vi "运维调试_五参数.vi"(11 "编号":string) -> ()   [LabVIEW 2016, in "斯坦道多参数.lvlib"]
uses:
  <vilib>/Utility/miscctls.llb/LVPointTypeDef.ctl
  <vilib>/Plasmionique/MB Master/MB_Master/MB_Master.lvclass
  <vilib>/Utility/config.llb/NI_LVConfig.lvlib
panel:
  in  "水样保存组数":dbl caption="水样保存组数:"
  in  "打开modbus":bool
  in  "仪器参数":bool
  in  "参数设置选项卡":enum32{"选项卡 1", "选项卡 2"}(tab)
  in  "pH":bool
  in  "DO":bool
  in  "Turb":bool
  in  "Cond":bool
  in  "Temp":bool
  in  "叶绿素a启用":bool
  in  "藻密度":bool
  in  "pH探头选择":u16(ring) items=["YL型", "MQ型", "NAQ型"]
  in  "DO探头选择":u16(ring) items=["YL型", "MQ型", "NAQ型"]
  in  "电导率探头选择":u16(ring) items=["YL型", "MQ型", "NAQ型"]
  in  "浊度探头选择":u16(ring) items=["YL型", "MQ型", "NAQ型"]
  in  "叶绿素a探头选择":u16(ring) items=["YL型", "MQ型", "NAQ型"]
  in  "藻密度探头选择":u16(ring) items=["YL型", "MQ型", "NAQ型"]
  in  "ORP启用":bool
  in  "ORP探头选择":u16(ring) items=["YL型", "MQ型", "NAQ型"]
  in  "校准选择":T1
  out "模块版本号":string
  out "权限等级":string
  in  "水样稳定时间":dbl caption="水样稳定时间:"
  out "选项卡控件":enum32{"选项卡 1", "选项卡 2"}(tab)
  in  "VISA资源名称":refnum<visa-resource-name> caption="串口"
  in  "电导率串口":refnum<visa-resource-name>
  in  "IP":string="localhost" caption="IP:"
  in  "Port":u16=502 caption="Port:"
  in  "自动断线重连":bool=TRUE
  in  "连接方式":u16(ring) items=["Modbus RTU", "Modbus TCP"]
  in  "密码锁":bool
  in  "设置页返回":bool
  in  "周期设置":bool
  out "当前串口":string
  out "运行状态":enum16{"空闲", "水样测试", "标样核查"}(ring)
  in  "停止":bool
  in  "标样核查":bool
  in  "水样测试":bool
  in  "设置":bool
  in  "探头校正返回":bool
  in  "探头校正":bool
  out "检测值":T2
  # "请设置仪器连接方式"
  # "组"
  # "请选择要启用的参数"
  # "min"
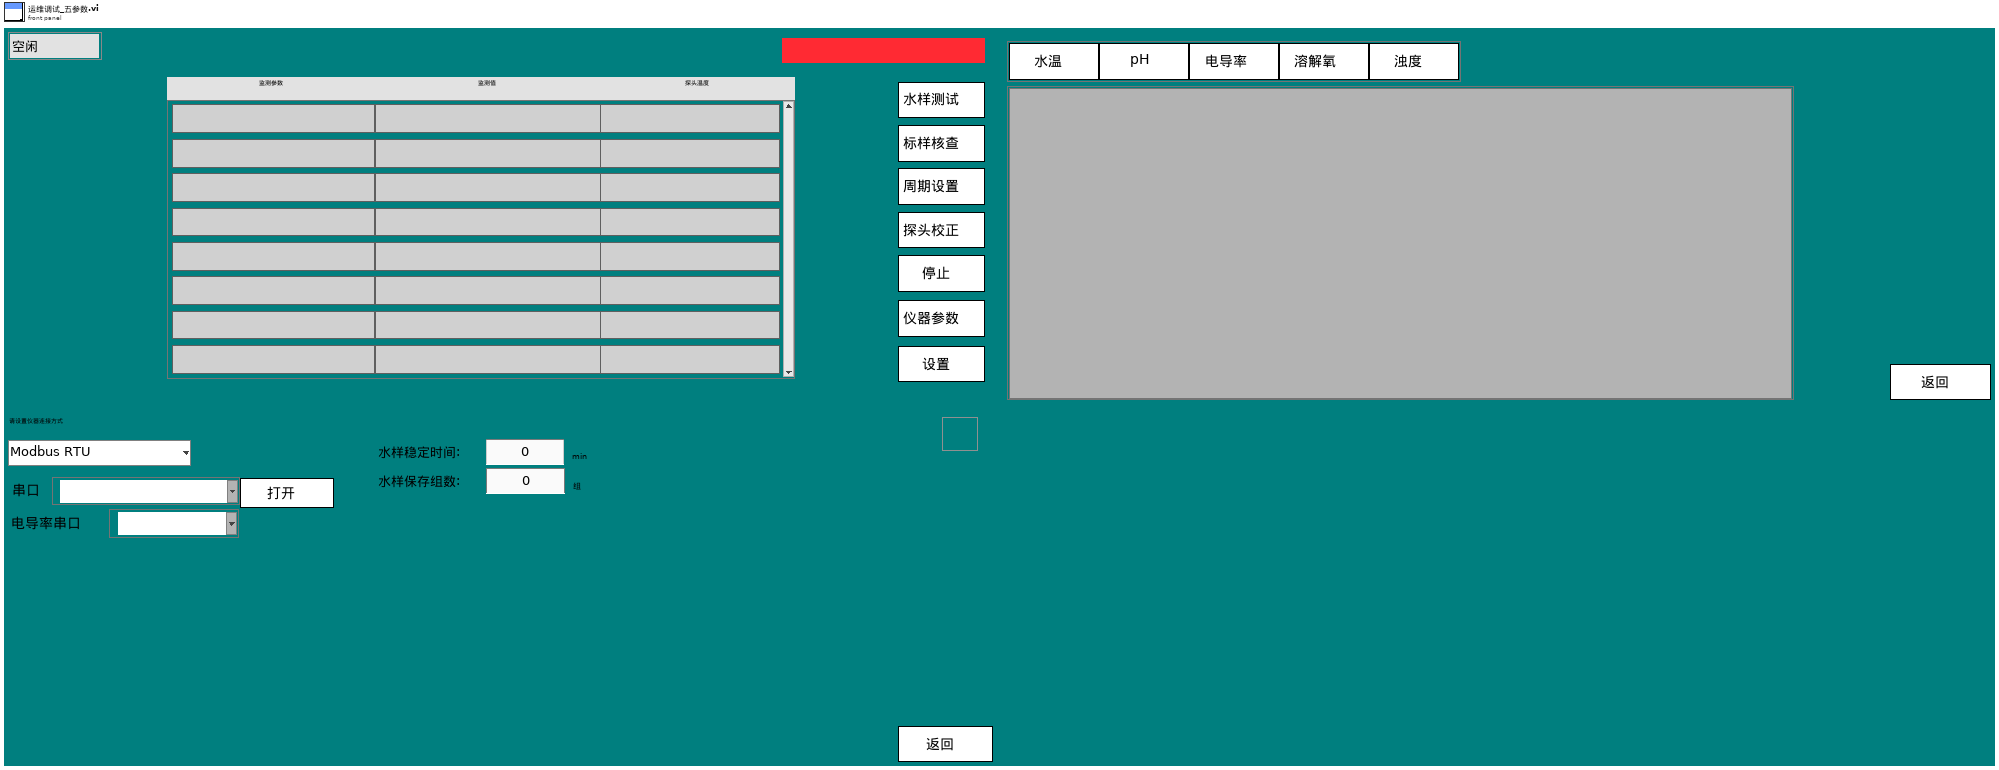
[diagram p1: front panel]
types:
  T1 = cluster{"水温校准":bool, "pH校准":bool, "电导率校准":bool, "溶解氧校准":bool, "浊度校准":bool, "叶绿素a校准":bool, "藻密度校准":bool, "ORP校准":bool}
  T2 = typedef "斯坦道多参数.lvlib/检测值.ctl" = cluster{"监测参数1":string, "浓度1":string, "探头温度1":string}[]
  T3 = typedef "LVPointTypeDef.ctl" = cluster{"Horizontal":i16, "Vertical":i16}
  T4 = cluster{"CH":u16, "监测值":dbl, "温度偏移修正值":sgl, "信号值":sgl}
  T5 = cluster{"温度测量值":sgl, "测量值":sgl, "温度偏移修正值":sgl, "信号值":sgl}
  T6 = cluster{"温度测量值":sgl, "DO%":sgl, "DOmg/L":sgl, "温度偏移修正值":sgl}
  T7 = cluster{"电极状态标志":u16, "电极型号标志":u16, "浊度测量值":sgl, "温度测量值":sgl, "浊度信号值":sgl, "浊度偏移修正值":sgl, "温度偏移修正值":sgl, "手动温度补偿值":sgl, "浊度电极零点":sgl, "浊度电极斜率":sgl, "第1点标准值记录":sgl, "第1点信号值记录":sgl, "第1点温度值记录":sgl, "第2点标准值记录":sgl, "第2点信号值记录":sgl, "第2点温度值记录":sgl, "命令滤波设定":u16, "温度模式":enum16{"ATC", "MTC"}, "生产批次":u16, "电极序号":u16, "串口地址":u16, "串口波特率":enum16{"9600", "19200", "115200"}, "串口校验位":enum16{"NONE", "ODD", "EVEN"}, "串口停止位":enum16{"1bit", "2bit"}, "第一点标准值":sgl, "第二点标准值":sgl, "第三点标准值":sgl}
  T8 = cluster{"电极状态标志":u16, "电极型号标志":u16, "溶解氧测量值":sgl, "温度测量值":sgl, "溶解氧饱和度值":sgl, "盐度补偿值":sgl, "大气压补偿值":sgl, "溶解氧偏移修正值":sgl, "温度偏移修正值":sgl, "手动温度补偿值":sgl, "溶解氧电极零点":sgl, "溶解氧电极斜率":sgl, "第1点标准值记录":sgl, "第1点信号值记录":sgl, "第1点温度值记录":sgl, "第2点标准值记录":sgl, "第2点信号值记录":sgl, "第2点温度值记录":sgl, "命令滤波设定":u16, "温度模式":enum16{"ATC", "MTC"}, "生产批次":u16, "电极序号":u16, "串口地址":u16, "串口波特率":enum16{"9600", "19200", "115200"}, "串口校验位":enum16{"NONE", "ODD", "EVEN"}, "串口停止位":enum16{"1bit", "2bit"}, "第一点标准值":sgl, "第二点标准值":sgl}
  T9 = cluster{"电极状态标志":u16, "电极型号标志":u16, "酸碱度测量值":sgl, "温度测量值":sgl, "酸碱度信号值":sgl, "温度信号值":sgl, "酸碱度偏移修正值":sgl, "温度偏移修正值":sgl, "手动温度补偿值":sgl, "酸碱度电极零点":sgl, "酸碱度电极斜率":sgl, "第1点标准值记录":sgl, "第1点信号值记录":sgl, "第1点温度值记录":sgl, "第2点标准值记录":sgl, "第2点信号值记录":sgl, "第2点温度值记录":sgl, "命令滤波设定":u16, "温度模式":enum16{"ATC", "MTC"}, "生产批次":u16, "电极序号":u16, "串口地址":u16, "串口波特率":enum16{"9600", "19200", "115200"}, "串口校验位":enum16{"NONE", "ODD", "EVEN"}, "串口停止位":enum16{"1bit", "2bit"}, "第一点标准值":sgl, "第二点标准值":sgl}
  T10 = cluster{"测量量程":dbl, "测量精度":dbl, "测量间隔":dbl, "消解温度":dbl, "消解时长":dbl, "空白校准时间":timestamp, "曲线截距":dbl, "曲线斜率":dbl, "测量检出限":dbl, "测量信号值":dbl, "线性相关系数":dbl, "二次多项式系数":dbl, "标样校准时间":timestamp, "稀释倍数":dbl, "三项式系数":dbl, "空白标定系数":dbl, "量程系数":dbl, "F0/ORPA":dbl, "F1/ORPB":dbl, "F2/ORPK":dbl, "F3":dbl, "F4":dbl, "F5":dbl, "F6":dbl, "F7":dbl, "X0/滴定数":dbl, "量程":dbl}
  T11 = cluster{"电极状态标志":u16, "电极型号标志":u16, "电导率测量值":sgl, "温度测量值":sgl, "电导率信号值":sgl, "温度信号值":sgl, "温度补偿系数":sgl, "电导率偏移修正值":sgl, "温度偏移修正值":sgl, "手动温度补偿值":sgl, "电导率电极零点":sgl, "电导率电极斜率":sgl, "命令滤波设定":u16, "温度模式":enum16{"ATC", "MTC"}, "生产批次":u16, "电极序号":u16, "串口地址":u16, "串口波特率":enum16{"9600", "19200", "115200"}, "串口校验位":enum16{"NONE", "ODD", "EVEN"}, "串口停止位":enum16{"1bit", "2bit"}, "第一点标准值":sgl, "第二点标准值":sgl}
  T12 = enum8{"Enabled", "Disabled", "Disabled and Grayed Out"}
  T13 = cluster{"pH探头选择":u16, "DO探头选择":u16, "电导率探头选择":u16, "浊度探头选择":u16, "叶绿素a探头选择":u16, "蓝绿藻探头选择":u16, "orp探头选择":u16}
  T14 = cluster{"监测参数1":string, "浓度1":string, "探头温度1":string}[]
  T15 = cluster{"周期设置类型":enum16{"定点启动", "间隔启动"}, "定时功能启用":bool, "定时间隔":u32, "24H周期设置":bool[]}
  T16 = enum32{"Bad", "Idle", "Run top level", "Running"}
  T17 = typedef "LVDateTimeRec.ctl" = cluster{"秒数的小数部分":dbl, "秒":i32, "分":i32, "时":i32, "日":i32, "月":i32, "年":i32, "天数（周）":i32, "天数（年）":i32, "DST":i32}
  T18 = cluster{"Major":u16, "Minor":u16, "Fix":u16, "Build":u16}
  T19 = typedef "NI_LVConfig.lvlib/Config Data RefNum.ctl" = refnum<k1>
  T20 = cluster{"baud rate (bps)":u32, "stop bits":u16, "parity":u16, "flow control":u16, "timeout":u32, "retries":i32}
  T21 = cluster{"pH校准VI引用句柄":refnum<vi>, "DO校准VI引用句柄":refnum<vi>, "COND校准VI引用句柄":refnum<vi>, "TURB校准VI引用句柄":refnum<vi>, "CHLA校准VI引用句柄":refnum<vi>, "BGA校准VI引用句柄":refnum<vi>, "ORP校准VI引用句柄":refnum<vi>}
  T22 = cluster{"测量量程":dbl, "测量精度":dbl, "测量间隔":dbl, "消解温度":dbl, "消解时长":dbl, "空白校准时间":timestamp, "曲线截距":dbl, "曲线斜率":dbl, "测量检出限":dbl, "测量信号值":dbl, "线性相关系数":dbl, "二次多项式系数":dbl, "标样校准时间":timestamp, "稀释倍数":dbl, "三项式系数":dbl, "空白标定系数":dbl, "量程系数":dbl, "F0/ORPA":dbl, "F1/ORPB":dbl, "F2/ORPK":dbl, "F3":dbl, "F4":dbl, "F5":dbl, "F6":dbl, "F7":dbl, "X0/滴定数":dbl, "量程":dbl}[]
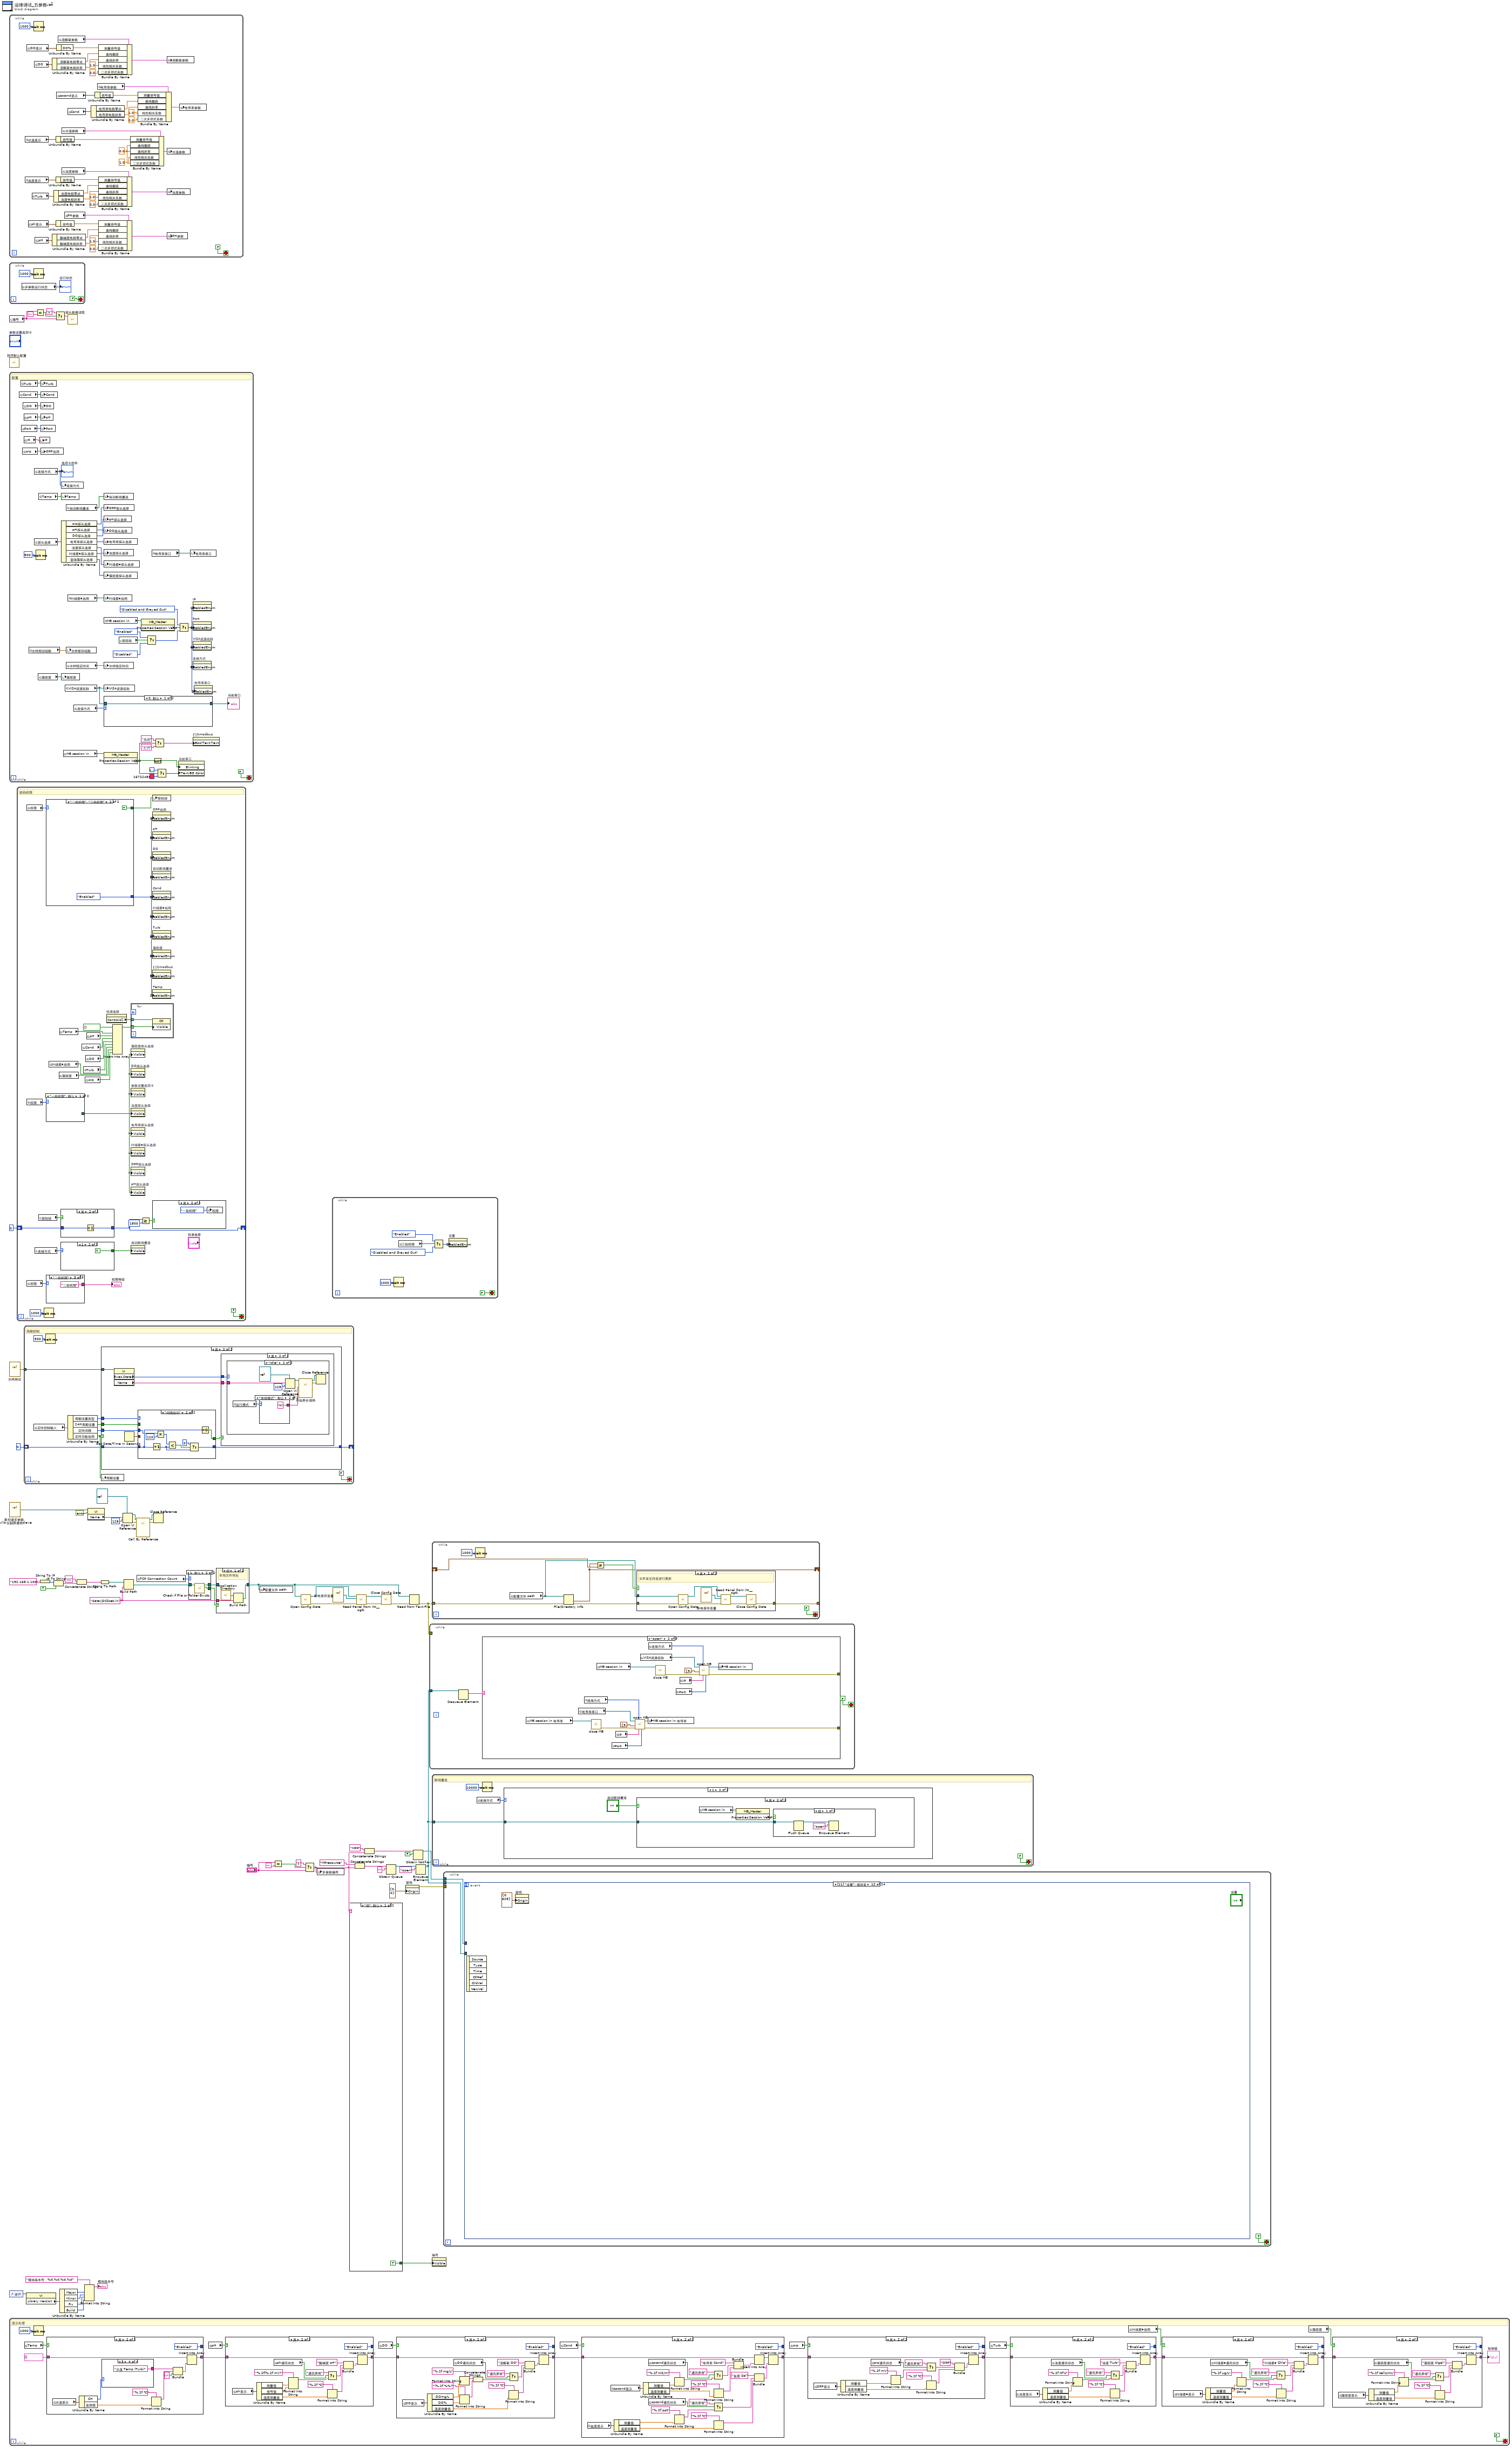
[diagram p0: block diagram]
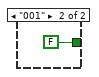
[diagram p3: hidden frame]
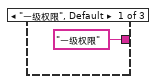
[diagram p12: hidden frame]
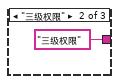
[diagram p13: hidden frame]
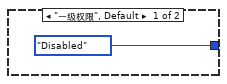
[diagram p14: hidden frame]
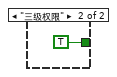
[diagram p15: hidden frame]
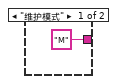
[diagram p19: hidden frame]
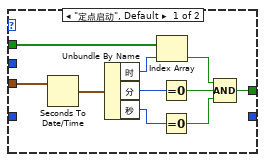
[diagram p20: hidden frame]
diagram:
  w34 = "data\\DCSset.ini" ("名称或相对路径")
  n1 = while {
    stop <- FALSE stop-if-true
    w64 = 0.0 ("二次多项式系数")
    n2 = global read "多参数全局变量.vi" "水温显示"() -> (w85:T4)
    n3 = global read "多参数全局变量.vi" "浊度显示"() -> (w67:T5)
    n4 = global read "多参数全局变量.vi" "DO显示"() -> (w99:T6)
    n5 = global read "多参数全局变量.vi" "ph显示"() -> (w94:T5)
    n6 = global read "国弘过程全局变量.vi" "Turb"() -> (w69:T7)
    n7 = Wait (ms)(milliseconds to wait=u32 1000 ("等待时间（毫秒）")) -> ()  [unwired: 1 out]
    n8 = global read "国弘过程全局变量.vi" "DO"() -> (w101:T8)
    n9 = global read "国弘过程全局变量.vi" "pH"() -> (w92:T9)
    n10 = Unbundle By Name(w101) -> ("溶解氧电极零点"=w102:sgl, "溶解氧电极斜率"=w103:sgl)
    n11 = Unbundle By Name(w92) -> ("酸碱度电极零点"=w91:sgl, "酸碱度电极斜率"=w90:sgl)
    n12 = Unbundle By Name(w69) -> ("浊度电极零点"=w70:sgl, "浊度电极斜率"=w71:sgl)
    n13 = Unbundle By Name(w85) -> ("信号值"=w86:sgl)
    n14 = Unbundle By Name(w67) -> ("信号值"=w68:sgl)
    n15 = Unbundle By Name(w94) -> ("信号值"=w93:sgl)
    n16 = Unbundle By Name(w99) -> ("DO%"=w100:sgl)
    n17 = global read "多参数全局变量.vi" "spcond显示"() -> (w80:T5)
    n18 = global read "断电保存变量.vi" "溶解氧参数"() -> (w97:T10)
    n19 = global read "断电保存变量.vi" "水温参数"() -> (w83:T10)
    n20 = global read "断电保存变量.vi" "浊度参数"() -> (w65:T10)
    n21 = global read "断电保存变量.vi" "PH参数"() -> (w96:T10)
    n22 = global read "国弘过程全局变量.vi" "Cond"() -> (w78:T11)
    n23 = Unbundle By Name(w78) -> ("电导率电极零点"=w77:sgl, "电导率电极斜率"=w76:sgl)
    n24 = Unbundle By Name(w80) -> ("信号值"=w79:sgl)
    n25 = global read "断电保存变量.vi" "电导率参数"() -> (w82:T10)
    n26 = Bundle By Name(cluster=w97, "测量信号值"=w100, "曲线截距"=w102, "曲线斜率"=w103, "线性相关系数"=1.0, "二次多项式系数"=0.0) -> (w98:T10)
    n27 = Bundle By Name(cluster=w65, "测量信号值"=w68, "曲线截距"=w70, "曲线斜率"=w71, "线性相关系数"=1.0, "二次多项式系数"=0.0) -> (w66:T10)
    n28 = Bundle By Name(cluster=w96, "测量信号值"=w93, "曲线截距"=w91, "曲线斜率"=w90, "线性相关系数"=1.0, "二次多项式系数"=0.0) -> (w95:T10)
    n29 = Bundle By Name(cluster=w83, "测量信号值"=w86, "曲线截距"=w64, "曲线斜率"=w64, "线性相关系数"=1.0, "二次多项式系数"=w64) -> (w84:T10)
    n30 = Bundle By Name(cluster=w82, "测量信号值"=w79, "曲线截距"=w77, "曲线斜率"=w76, "线性相关系数"=1.0, "二次多项式系数"=0.0) -> (w81:T10)
    n31 = global write "断电保存变量.vi" "溶解氧参数"(w98) -> ()
    n32 = global write "断电保存变量.vi" "水温参数"(w84) -> ()
    n33 = global write "断电保存变量.vi" "浊度参数"(w66) -> ()
    n34 = global write "断电保存变量.vi" "PH参数"(w95) -> ()
    n35 = global write "断电保存变量.vi" "电导率参数"(w81) -> ()
  }
  n36 = while {
    stop <- FALSE stop-if-true
    n37 = global read "多参数全局变量.vi" "多参数运行状态"() -> (→"运行状态":u16)
    n38 = Wait (ms)(milliseconds to wait=u32 1000 ("等待时间（毫秒）")) -> ()  [unwired: 1 out]
  }
  n39 = local read "编号"() -> (w10:string)
  n40 = call "程序默认配置.vi"() -> ()  [unwired: 11 in, 1 out]
  n41 = while {
    stop <- FALSE stop-if-true
    # "配置"
    n42 = global read "断电保存变量.vi" "Cond"() -> (w151:bool)
    n43 = global read "断电保存变量.vi" "Turb"() -> (w150:bool)
    n44 = global read "断电保存变量.vi" "Port"() -> (w129:u16)
    n45 = global read "断电保存变量.vi" "orp"() -> (w115:bool)
    n46 = global read "断电保存变量.vi" "DO"() -> (w152:bool)
    n47 = global read "断电保存变量.vi" "pH"() -> (w153:bool)
    n48 = global read "断电保存变量.vi" "IP"() -> (w130:string)
    n49 = global read "断电保存变量.vi" "水样测试组数"() -> (w111:dbl)
    n50 = global read "断电保存变量.vi" "连接方式"() -> (w123:u16)
    "选项卡控件" <- w123
    n51 = global read "断电保存变量.vi" "探头选择"() -> (w140:T13)
    n52 = Wait (ms)(milliseconds to wait=u32 500 ("等待时间（毫秒）")) -> ()  [unwired: 1 out]
    n53 = global read "断电保存变量.vi" "藻密度"() -> (w148:bool)
    n54 = global read "断电保存变量.vi" "Temp"() -> (w154:bool)
    n55 = local write "IP"(w130) -> ()
    n56 = local write "Turb"(w150) -> ()
    n57 = local write "Cond"(w151) -> ()
    n58 = local write "DO"(w152) -> ()
    n59 = local write "pH"(w153) -> ()
    n60 = local write "Port"(w129) -> ()
    n61 = local write "ORP启用"(w115) -> ()
    n62 = local write "连接方式"(w123) -> ()
    n63 = local write "Temp"(w154) -> ()
    n64 = Unbundle By Name(w140) -> ("orp探头选择"=w114:u16, "pH探头选择"=w124:u16, "DO探头选择"=w139:u16, "电导率探头选择"=w138:u16, "浊度探头选择"=w137:u16, "叶绿素a探头选择"=w136:u16, "蓝绿藻探头选择"=w135:u16)
    n65 = local write "藻密度"(w148) -> ()
    n66 = global read "多参数全局变量.vi" "MB session in"() -> (w144:refnum<class "MB_Master.lvclass">)
    n67 = global read "断电保存变量.vi" "VISA资源名称"() -> (w127:refnum<visa-resource-name>)
    n68 = global read "断电保存变量.vi" "自动断线重连"() -> (w118:bool)
    n69 = local write "水样保存组数"(w111) -> ()
    n70 = global read "断电保存变量.vi" "水样稳定时间"() -> (w117:dbl)
    n71 = global read "断电保存变量.vi" "叶绿素a启用"() -> (w149:bool)
    n72 = global read "断电保存变量.vi" "连接方式"() -> (w128:u16)
    n73 = local write "自动断线重连"(w118) -> ()
    n74 = local write "ORP探头选择"(w114) -> ()
    n75 = local write "pH探头选择"(w124) -> ()
    n76 = local write "DO探头选择"(w139) -> ()
    n77 = local write "电导率探头选择"(w138) -> ()
    n78 = local write "浊度探头选择"(w137) -> ()
    n79 = local write "叶绿素a探头选择"(w136) -> ()
    n80 = local write "藻密度探头选择"(w135) -> ()
    n81 = local write "叶绿素a启用"(w149) -> ()
    n82 = global read "多参数全局变量.vi" "MB session in"() -> (w147:refnum<class "MB_Master.lvclass">)
    n83 = local write "水样稳定时间"(w117) -> ()
    n84 = local write "VISA资源名称"(w127) -> ()
    n85 = case shown="0, 默认" w128 {
      tunnel: w127 -> [w156 _]
      tunnel: [w156 w157] -> w126
      frame 0, Default {
      }
      frame 1 {
        n86 = global read "断电保存变量.vi" "Port"() -> (w158:u16)
        n87 = global read "断电保存变量.vi" "IP"() -> (w160:string)
        n88 = Format Into String(format string=":%d" ("格式字符串"), initial string=w160, w158) -> (resulting string=w157:string)  [unwired: 1 in, 1 out]
      }
    }
    "当前串口" <- w126
    n89 = property class="MB_Master"(reference=w144) -> ("Properties:Session Valid"=w122:bool)  [unwired: 1 in, 2 out]
    n90 = local read "密码锁"() -> (w134:bool)
    n91 = property class="MB_Master"(reference=w147) -> ("Properties:Session Valid"=w146:bool)  [unwired: 1 in, 2 out]
    n92 = Select(t=T12."Enabled" ("f"), s=w134, f=T12."Disabled") -> (s? t:f=w132:T12)
    n93 = global read "断电保存变量.vi" "电导率串口"() -> (w112:refnum<visa-resource-name>)
    n94 = Not(x=w122) -> (.not. x?=w125:bool)
    n95 = Select(t="关闭" ("布尔文本.文本"), s=w122, f="打开" ("布尔文本.文本")) -> (s? t:f=w141:string)
    n96 = Select(t=u32 16777216, s=w122, f=u32 16722483) -> (s? t:f=w119:u32)
    n97 = property on="当前串口" class="Str"("Blinking"=w125, "Text.BG Color"=w119) -> ()  [unwired: 2 in, 2 out]
    n98 = Select(t=T12."Disabled and Grayed Out" ("禁用"), s=w146, f=w132) -> (s? t:f=w113:T12)
    n99 = local write "电导率串口"(w112) -> ()
    n100 = property on="IP" class="Str"("DisabledEnum"=w113) -> ()  [unwired: 2 in, 2 out]
    n101 = property on="Port" class="DigNum (严格)"("DisabledEnum"=w113) -> ()  [unwired: 2 in, 2 out]
    n102 = property on="VISA资源名称" class="VISAName"("DisabledEnum"=w113) -> ()  [unwired: 2 in, 2 out]
    n103 = property on="连接方式" class="Ring (严格)"("DisabledEnum"=w113) -> ()  [unwired: 2 in, 2 out]
    n104 = property on="打开modbus" class="Bool"("BoolText.Text"=w141) -> ()  [unwired: 2 in, 2 out]
    n105 = property on="电导率串口" class="VISAName"("DisabledEnum"=w113) -> ()  [unwired: 2 in, 2 out]
  }
  n106 = vi-ref "水样测试.vi"() -> (w53:refnum<vi>)
  n107 = vi-ref "斯坦道多参数.lvlib:主副屏通信slave.vi"() -> (w35:refnum<vi>)
  n108 = control-ref of="本VI"() -> (w26:refnum<vi>)
  n109 = while {
    stop <- FALSE stop-if-true
    # "显示处理"
    n110 = global read "断电保存变量.vi" "Temp"() -> (w177:bool)
    n111 = Wait (ms)(milliseconds to wait=u32 1000 ("等待时间（毫秒）")) -> ()  [unwired: 1 out]
    n112 = case shown="真" w177 {
      tunnel: [w318 w323] -> w174
      tunnel: T14 [] ("数组") -> [w318 w324]
      tunnel: [T12."Disabled and Grayed Out" ("禁用") T12."Enabled" ("禁用")] -> _
      frame False {
      }
      frame True {
        n113 = global read "多参数全局变量.vi" "水温显示"() -> (w321:T4)
        n114 = Unbundle By Name(w321) -> ("CH"=w320:u16, "监测值"=w319:dbl)
        n115 = case shown="3" w320 {
          tunnel: ["水温 Temp (pH)" ("监测参数1") "水温 Temp (Cond)" ("监测参数1") "水温 Temp (DO)" ("监测参数1") "水温 Temp (Turb)" ("监测参数1")] -> w328
          frame 0, Default {
          }
          frame 1 {
          }
          frame 2 {
          }
          frame 3 {
          }
        }
        n116 = Format Into String(format string="%.2f ℃" ("格式字符串"), w319) -> (resulting string=w327:string)  [unwired: 2 in, 1 out]
        n117 = Bundle("监测参数1"=w328, w327, "探头温度1"="-") -> (w325:cluster{"监测参数1":string, string, "探头温度1":string})  [unwired: 1 in]
        n118 = Insert Into Array(array=w324, new element=w325) -> (w323:T14)  [unwired: 1 in]
      }
    }
    n119 = global read "断电保存变量.vi" "pH"() -> (w175:bool)
    n120 = case shown="真" w175 {
      tunnel: [w300 w308] -> w172
      tunnel: w174 -> [w300 w310]
      tunnel: [T12."Disabled and Grayed Out" ("禁用") T12."Enabled" ("禁用")] -> _
      frame False {
      }
      frame True {
        n121 = global read "多参数全局变量.vi" "ph显示"() -> (w306:T5)
        n122 = Unbundle By Name(w306) -> ("测量值"=w316:sgl, "信号值"=w301:sgl, "温度测量值"=w314:sgl)
        n123 = global read "多参数全局变量.vi" "ph通讯状态"() -> (w304:bool)
        n124 = Format Into String(format string="%.2f(%.2f mV)" ("格式字符串"), w316, w301) -> (resulting string=w303:string)  [unwired: 2 in, 1 out]
        n125 = Select(t="通讯异常" ("格式字符串"), s=w304, f=w303) -> (s? t:f=w302:string)
        n126 = Format Into String(format string="%.2f ℃" ("格式字符串"), w314) -> (resulting string=w312:string)  [unwired: 2 in, 1 out]
        n127 = Bundle("监测参数2"="酸碱度 pH", "格式字符串"=w302, w312) -> (w309:cluster{"监测参数2":string, "格式字符串":string, string})  [unwired: 1 in]
        n128 = Insert Into Array(array=w310, new element=w309) -> (w308:T14)  [unwired: 1 in]
      }
    }
    n129 = global read "断电保存变量.vi" "DO"() -> (w173:bool)
    n130 = case shown="真" w173 {
      tunnel: [w279 w286] -> w169
      tunnel: w172 -> [w279 w287]
      tunnel: [T12."Disabled and Grayed Out" ("禁用") T12."Enabled" ("禁用")] -> _
      frame False {
      }
      frame True {
        n131 = global read "多参数全局变量.vi" "DO显示"() -> (w284:T6)
        n132 = Unbundle By Name(w284) -> ("DOmg/L"=w295:sgl, "DO%"=w293:sgl, "温度测量值"=w297:sgl)
        n133 = global read "多参数全局变量.vi" "DO通讯状态"() -> (w282:bool)
        n134 = Format Into String(format string="%.2f mg/L" ("格式字符串"), w295) -> (resulting string=w292:string)  [unwired: 2 in, 1 out]
        n135 = Format Into String(format string="(%.2f %%)" ("格式字符串"), w293) -> (resulting string=w291:string)  [unwired: 2 in, 1 out]
        n136 = Concatenate Strings(w292, w291) -> (w281:string)
        n137 = Select(t="通讯异常" ("格式字符串"), s=w282, f=w281) -> (s? t:f=w280:string)
        n138 = Format Into String(format string="%.2f ℃" ("格式字符串"), w297) -> (resulting string=w289:string)  [unwired: 2 in, 1 out]
        n139 = Bundle("监测参数2"="溶解氧 DO", "格式字符串"=w280, w289) -> (w288:cluster{"监测参数2":string, "格式字符串":string, string})  [unwired: 1 in]
        n140 = Insert Into Array(array=w287, new element=w288) -> (w286:T14)  [unwired: 1 in]
      }
    }
    n141 = global read "断电保存变量.vi" "Cond"() -> (w171:bool)
    n142 = case shown="真" w171 {
      tunnel: w169 -> [w249 w273]
      tunnel: [w249 w262] -> w161
      tunnel: [T12."Disabled and Grayed Out" ("禁用") T12."Enabled" ("禁用")] -> _
      frame False {
      }
      frame True {
        n143 = global read "多参数全局变量.vi" "盐度显示"() -> (w255:T5)
        n144 = global read "多参数全局变量.vi" "spcond显示"() -> (w270:T5)
        n145 = Unbundle By Name(w255) -> ("测量值"=w256:sgl, "温度测量值"=w257:sgl)
        n146 = Unbundle By Name(w270) -> ("测量值"=w269:sgl, "温度测量值"=w268:sgl)
        n147 = global read "多参数全局变量.vi" "spcond通讯状态"() -> (w266:bool)
        n148 = global read "多参数全局变量.vi" "spcond通讯状态"() -> (w259:bool)
        n149 = Format Into String(format string="%.2f mS/m" ("格式字符串"), w269) -> (resulting string=w265:string)  [unwired: 2 in, 1 out]
        n150 = Format Into String(format string="%.2f ppt" ("格式字符串"), w256) -> (resulting string=w260:string)  [unwired: 2 in, 1 out]
        n151 = Select(t="通讯异常" ("格式字符串"), s=w266, f=w265) -> (s? t:f=w264:string)
        n152 = Select(t="通讯异常" ("格式字符串"), s=w259, f=w260) -> (s? t:f=w261:string)
        n153 = Format Into String(format string="%.2f ℃" ("格式字符串"), w268) -> (resulting string=w274:string)  [unwired: 2 in, 1 out]
        n154 = Format Into String(format string="%.2f ℃" ("格式字符串"), w257) -> (resulting string=w254:string)  [unwired: 2 in, 1 out]
        n155 = Bundle("监测参数2"="电导率 Cond", "格式字符串"=w264, w274) -> (w272:cluster{"监测参数2":string, "格式字符串":string, string})  [unwired: 1 in]
        n156 = Insert Into Array(array=w273, new element=w272) -> (w263:T14)  [unwired: 1 in]
        n157 = Bundle("监测参数2"="盐度 Sal", "格式字符串"=w261, w254) -> (w250:cluster{"监测参数2":string, "格式字符串":string, string})  [unwired: 1 in]
        n158 = Insert Into Array(array=w263, new element=w250) -> (w262:T14)  [unwired: 1 in]
      }
    }
    n159 = global read "断电保存变量.vi" "orp"() -> (w163:bool)
    n160 = case shown="真" w163 {
      tunnel: w161 -> [w181 w192]
      tunnel: [w181 w190] -> w162
      tunnel: [T12."Disabled and Grayed Out" ("禁用") T12."Enabled" ("禁用")] -> _
      frame False {
      }
      frame True {
        n161 = global read "多参数全局变量.vi" "ORP显示"() -> (w188:T5)
        n162 = Unbundle By Name(w188) -> ("测量值"=w187:sgl, "温度测量值"=w186:sgl)
        n163 = global read "多参数全局变量.vi" "orp通讯状态"() -> (w184:bool)
        n164 = Format Into String(format string="%.2f mV" ("格式字符串"), w187) -> (resulting string=w183:string)  [unwired: 2 in, 1 out]
        n165 = Select(t="通讯异常" ("格式字符串"), s=w184, f=w183) -> (s? t:f=w182:string)
        n166 = Format Into String(format string="%.2f ℃" ("格式字符串"), w186) -> (resulting string=w193:string)  [unwired: 2 in, 1 out]
        n167 = Bundle("监测参数2"="ORP", "格式字符串"=w182, w193) -> (w191:cluster{"监测参数2":string, "格式字符串":string, string})  [unwired: 1 in]
        n168 = Insert Into Array(array=w192, new element=w191) -> (w190:T14)  [unwired: 1 in]
      }
    }
    n169 = global read "断电保存变量.vi" "Turb"() -> (w170:bool)
    n170 = case shown="真" w170 {
      tunnel: w162 -> [w232 w243]
      tunnel: [w232 w241] -> w168
      tunnel: [T12."Disabled and Grayed Out" ("禁用") T12."Enabled" ("禁用")] -> _
      frame False {
      }
      frame True {
        n171 = global read "多参数全局变量.vi" "浊度显示"() -> (w239:T5)
        n172 = Unbundle By Name(w239) -> ("测量值"=w238:sgl, "温度测量值"=w237:sgl)
        n173 = global read "多参数全局变量.vi" "浊度通讯状态"() -> (w235:bool)
        n174 = Format Into String(format string="%.2f NTU" ("格式字符串"), w238) -> (resulting string=w234:string)  [unwired: 2 in, 1 out]
        n175 = Select(t="通讯异常" ("格式字符串"), s=w235, f=w234) -> (s? t:f=w233:string)
        n176 = Format Into String(format string="%.2f ℃" ("格式字符串"), w237) -> (resulting string=w245:string)  [unwired: 2 in, 1 out]
        n177 = Bundle("监测参数2"="浊度 Turb", "格式字符串"=w233, w245) -> (w242:cluster{"监测参数2":string, "格式字符串":string, string})  [unwired: 1 in]
        n178 = Insert Into Array(array=w243, new element=w242) -> (w241:T14)  [unwired: 1 in]
      }
    }
    n179 = global read "断电保存变量.vi" "叶绿素a启用"() -> (w167:bool)
    n180 = case shown="真" w167 {
      tunnel: w168 -> [w215 w226]
      tunnel: [w215 w224] -> w165
      tunnel: [T12."Disabled and Grayed Out" ("禁用") T12."Enabled" ("禁用")] -> _
      frame False {
      }
      frame True {
        n181 = global read "多参数全局变量.vi" "叶绿素a显示"() -> (w220:T5)
        n182 = Unbundle By Name(w220) -> ("测量值"=w223:sgl, "温度测量值"=w222:sgl)
        n183 = global read "多参数全局变量.vi" "叶绿素a通讯状态"() -> (w218:bool)
        n184 = Format Into String(format string="%.2f μg/L" ("格式字符串"), w223) -> (resulting string=w217:string)  [unwired: 2 in, 1 out]
        n185 = Select(t="通讯异常" ("格式字符串"), s=w218, f=w217) -> (s? t:f=w216:string)
        n186 = Format Into String(format string="%.2f ℃" ("格式字符串"), w222) -> (resulting string=w228:string)  [unwired: 2 in, 1 out]
        n187 = Bundle("监测参数2"="叶绿素a Chla", "格式字符串"=w216, w228) -> (w225:cluster{"监测参数2":string, "格式字符串":string, string})  [unwired: 1 in]
        n188 = Insert Into Array(array=w226, new element=w225) -> (w224:T14)  [unwired: 1 in]
      }
    }
    n189 = global read "断电保存变量.vi" "藻密度"() -> (w166:bool)
    n190 = case shown="真" w166 {
      tunnel: w165 -> [w198 w209]
      tunnel: [w198 w207] -> w164
      tunnel: [T12."Disabled and Grayed Out" ("禁用") T12."Enabled" ("禁用")] -> _
      frame False {
      }
      frame True {
        n191 = global read "多参数全局变量.vi" "藻密度显示"() -> (w203:T5)
        n192 = Unbundle By Name(w203) -> ("测量值"=w206:sgl, "温度测量值"=w205:sgl)
        n193 = global read "多参数全局变量.vi" "藻密度通讯状态"() -> (w201:bool)
        n194 = Format Into String(format string="%.2f cells/mL" ("格式字符串"), w206) -> (resulting string=w200:string)  [unwired: 2 in, 1 out]
        n195 = Select(t="通讯异常" ("格式字符串"), s=w201, f=w200) -> (s? t:f=w199:string)
        n196 = Format Into String(format string="%.2f ℃" ("格式字符串"), w205) -> (resulting string=w211:string)  [unwired: 2 in, 1 out]
        n197 = Bundle("监测参数2"="藻密度 Algal", "格式字符串"=w199, w211) -> (w208:cluster{"监测参数2":string, "格式字符串":string, string})  [unwired: 1 in]
        n198 = Insert Into Array(array=w209, new element=w208) -> (w207:T14)  [unwired: 1 in]
      }
    }
    "检测值" <- w164
  }
  n199 = while {
    shift-right: [w356] -> _
    shift-left: u32 0 ("等待时间（毫秒）") -> [w357]
    stop <- FALSE stop-if-true
    # "密码权限"
    n200 = global read "多参数全局变量.vi" "权限"() -> (w347:enum16{"一级权限", "二级权限", "三级权限"})
    n201 = global read "多参数全局变量.vi" "权限"() -> (w348:enum16{"一级权限", "二级权限", "三级权限"})
    n202 = global read "多参数全局变量.vi" "权限"() -> (w349:enum16{"一级权限", "二级权限", "三级权限"})
    n203 = local read "连接方式"() -> (w353:u16)
    n204 = local read "密码锁"() -> (w358:bool)
    n205 = Wait (ms)(milliseconds to wait=u32 1000 ("等待时间（毫秒）")) -> ()  [unwired: 1 out]
    n206 = case shown="\"二级权限\", \"三级权限\"" w347 {
      tunnel: [T12."Disabled" ("禁用") T12."Enabled" ("禁用")] -> w351
      tunnel: [_ TRUE ("可见")] -> w346
      frame "一级权限", Default {
      }
      frame "二级权限", "三级权限" {
      }
    }
    n207 = case shown="\"一级权限\", 默认" w348 {
      tunnel: [_ TRUE ("可见")] -> w334
      frame "一级权限", Default {
      }
      frame "三级权限" {
      }
    }
    n208 = case shown="\"二级权限\"" w349 {
      tunnel: ["一级权限" ("权限等级") "三级权限" ("权限等级") "二级权限" ("权限等级")] -> w350
      frame "一级权限", Default {
      }
      frame "三级权限" {
      }
      frame "二级权限" {
      }
    }
    "权限等级" <- w350
    n209 = global read "断电保存变量.vi" "叶绿素a启用"() -> (w338:bool)
    n210 = global read "断电保存变量.vi" "藻密度"() -> (w337:bool)
    n211 = global read "断电保存变量.vi" "Temp"() -> (w344:bool)
    n212 = case shown="真" w358 {
      tunnel: w357 -> [_ w366]
      tunnel: [_ w365] -> w356
      frame False {
      }
      frame True {
        n213 = Increment(x=w366) -> (x+1=w365:u32)
      }
    }
    n214 = case shown="1" w353 {
      tunnel: [_ TRUE ("可见")] -> w352
      frame 0, Default {
      }
      frame 1 {
      }
    }
    n215 = global read "断电保存变量.vi" "Cond"() -> (w341:bool)
    n216 = global read "断电保存变量.vi" "Turb"() -> (w339:bool)
    n217 = global read "断电保存变量.vi" "orp"() -> (w336:bool)
    n218 = global read "断电保存变量.vi" "DO"() -> (w340:bool)
    n219 = global read "断电保存变量.vi" "pH"() -> (w342:bool)
    n220 = property on="校准选择" class="Clust"() -> ("Controls[]"=w345:refnum<vi>[])  [unwired: 2 in, 2 out]
    n221 = Insert Into Array(array=bool[] [] ("数组"), new element #1=w344, new element #2=w342, new element #3=w341, new element #4=w340, new element #5=w339, new element #6=w338, new element #7=w337, new element #8=w336) -> (w335:bool[])  [unwired: 1 in]
    n222 = for {
      tunnel: w345 -> [w362] mode=indexing
      tunnel: w335 -> [w361] mode=indexing
      n223 = property class="Ctl"(reference=w362, "Visible"=w361) -> ()  [unwired: 1 in, 2 out]
    }
    n224 = property on="藻密度探头选择" class="Ring (严格)"("Visible"=w334) -> ()  [unwired: 2 in, 2 out]
    n225 = property on="DO探头选择" class="Ring (严格)"("Visible"=w334) -> ()  [unwired: 2 in, 2 out]
    n226 = property on="参数设置选项卡" class="TabCtl (严格)"("Visible"=w334) -> ()  [unwired: 2 in, 2 out]
    n227 = property on="浊度探头选择" class="Ring (严格)"("Visible"=w334) -> ()  [unwired: 2 in, 2 out]
    n228 = property on="电导率探头选择" class="Ring (严格)"("Visible"=w334) -> ()  [unwired: 2 in, 2 out]
    n229 = property on="叶绿素a探头选择" class="Ring (严格)"("Visible"=w334) -> ()  [unwired: 2 in, 2 out]
    n230 = property on="ORP探头选择" class="Ring (严格)"("Visible"=w334) -> ()  [unwired: 2 in, 2 out]
    n231 = property on="pH探头选择" class="Ring (严格)"("Visible"=w334) -> ()  [unwired: 2 in, 2 out]
    n232 = property on="自动断线重连" class="Bool (严格)"("Visible"=w352) -> ()  [unwired: 2 in, 2 out]
    n233 = Greater Or Equal?(x=w356, y=u32 1800) -> (x >= y?=w354:bool)
    n234 = local write "密码锁"(w346) -> ()
    n235 = property on="ORP启用" class="Bool (严格)"("DisabledEnum"=w351) -> ()  [unwired: 2 in, 2 out]
    n236 = property on="pH" class="Bool (严格)"("DisabledEnum"=w351) -> ()  [unwired: 2 in, 2 out]
    n237 = property on="DO" class="Bool (严格)"("DisabledEnum"=w351) -> ()  [unwired: 2 in, 2 out]
    n238 = property on="自动断线重连" class="Bool (严格)"("DisabledEnum"=w351) -> ()  [unwired: 2 in, 2 out]
    n239 = property on="Cond" class="Bool (严格)"("DisabledEnum"=w351) -> ()  [unwired: 2 in, 2 out]
    n240 = property on="叶绿素a启用" class="Bool (严格)"("DisabledEnum"=w351) -> ()  [unwired: 2 in, 2 out]
    n241 = property on="Turb" class="Bool (严格)"("DisabledEnum"=w351) -> ()  [unwired: 2 in, 2 out]
    n242 = property on="藻密度" class="Bool (严格)"("DisabledEnum"=w351) -> ()  [unwired: 2 in, 2 out]
    n243 = property on="打开modbus" class="Bool"("DisabledEnum"=w351) -> ()  [unwired: 2 in, 2 out]
    n244 = property on="Temp" class="Bool (严格)"("DisabledEnum"=w351) -> ()  [unwired: 2 in, 2 out]
    n245 = case shown="真" w354 {
      frame False {
      }
      frame True {
        n246 = global write "多参数全局变量.vi" "权限"(enum16{"一级权限", "二级权限", "三级权限"}."一级权限" ("权限")) -> ()
      }
    }
  }
  n247 = while {
    tunnel: w53 -> [w376]
    shift-right: [w375] -> _
    shift-left: u32 0 ("等待时间（毫秒）") -> [w377]
    stop <- FALSE stop-if-true
    # "周期控制"
    n248 = global read "断电保存变量.vi" "定时控制输入"() -> (w379:T15)
    n249 = Wait (ms)(milliseconds to wait=u32 500 ("等待时间（毫秒）")) -> ()  [unwired: 1 out]
    n250 = Unbundle By Name(w379) -> ("周期设置类型"=w381:enum16{"定点启动", "间隔启动"}, "24H周期设置"=w380:bool[], "定时间隔"=w378:u32, "定时功能启用"=w374:bool)
    n251 = case shown="真" w374 {
      tunnel: w381 -> [_ w392]
      tunnel: w380 -> [_ w391]
      tunnel: w378 -> [_ w389]
      tunnel: w377 -> [_ w385]
      tunnel: w376 -> [_ w388]
      tunnel: [_ w384] -> w375
      frame False {
      }
      frame True {
        n252 = property class="VI"(reference=w388) -> ("Exec.State"=w386:T16, "Name"=w387:string)  [unwired: 1 in, 2 out]
        n253 = Get Date/Time In Seconds() -> (seconds since 1Jan1904=w393:timestamp)
        n254 = case shown="\"间隔启动\"" w392 {
          tunnel: w393 -> [w415 _]
          tunnel: w391 -> [w412 _]
          tunnel: [w406 w423] -> w390
          tunnel: w389 -> [_ w422]
          tunnel: w385 -> [_ w424]
          tunnel: [_ w418] -> w384
          frame "定点启动", Default {
            n255 = Seconds To Date/Time(time stamp (now)=w415) -> (date time rec=w414:T17)  [unwired: 1 in]
            n256 = Unbundle By Name(w414) -> ("时"=w413:i32, "分"=w411:i32, "秒"=w410:i32)
            n257 = Index Array(array=w412, index=w413) -> (element=w409:bool)
            n258 = Equal To 0?(x=w411) -> (x = 0?=w408:bool)
            n259 = Equal To 0?(x=w410) -> (x = 0?=w407:bool)
            n260 = Compound Arithmetic op=AND ("复合运算")(w409, w408, w407) -> (w406:bool)
          }
          frame "间隔启动" {
            n261 = Increment(x=w424) -> (x+1=w417:u32)
            n262 = Multiply(x=w422, y=u32 120) -> (x*y=w416:u32)
            n263 = Less?(x=w416, y=w417) -> (x < y?=w420:bool)
            n264 = Select(t=u32 0 ("y"), s=w420, f=w417) -> (s? t:f=w418:u32)
            n265 = Equal To 0?(x=w424) -> (x = 0?=w423:bool)
          }
        }
        n266 = case shown="真" w390 {
          tunnel: w386 -> [_ w395]
          tunnel: w387 -> [_ w394]
          frame False {
          }
          frame True {
            n267 = case shown="\"Idle\"" w395 {
              tunnel: w394 -> [_ w400]
              frame "Bad", Default {
              }
              frame "Idle" {
                n268 = global read "多参数全局变量.vi" "运行模式"() -> (w398:enum16{"维护模式", "常规模式", "应急模式", "质控模式"})
                n269 = case shown="\"常规模式\", 默认" w398 {
                  tunnel: ["M" ("数据标记表") "N" ("数据标记表")] -> w397
                  frame "维护模式" {
                  }
                  frame "常规模式", Default {
                  }
                }
                n270 = Open VI Reference(type specifier VI Refnum (for type only)=refnum<vi> refnum, vi path=w400, options=128 ("选项")) -> (vi reference=w401:refnum<vi>)  [unwired: 3 in, 1 out]
                n271 = call-by-ref "开始异步调用"(reference=w401, "数据标记表"=w397) -> (reference out=w402:refnum<vi>, error out=w403:errorcluster)  [unwired: 12 in]
                n272 = Close Reference(reference=w402, error in (no error)=w403) -> ()  [unwired: 1 out]
              }
            }
          }
        }
      }
    }
    n273 = local write "周期设置"(w374) -> ()
  }
  n274 = property class="VI"(reference=w26) -> ("Library.Version"=w25:T18)  [unwired: 1 in, 2 out]
  n275 = Equal?(x=w10, y="") -> (x = y?=w12:bool)
  n276 = String To IP(1:"192.168.1.100" ("名称")) -> (0:w33:u32)
  n277 = IP To String(1:TRUE ("句点符号？(F)"), 2:w33) -> (0:w30:string)
  n278 = Select(t="1", s=w12, f=w10) -> (s? t:f=w9:string)
  n279 = Unbundle By Name(w25) -> ("Major"=w23:u16, "Minor"=w22:u16, "Fix"=w21:u16, "Build"=w20:u16)
  n280 = call "探头数据读取.vi"("编号"=w9) -> ()  [unwired: 11 in]
  n281 = Concatenate Strings("\\\\" ("字符串"), w30) -> (w31:string)
  n282 = Format Into String(format string="模块版本号：%d.%d.%d.%d" ("格式字符串"), w23, w22, w21, w20) -> (resulting string=→"模块版本号":string)  [unwired: 2 in, 1 out]
  n283 = property class="VI"(reference=w35, error in=errorcluster {"status"=FALSE, "code"=0, "source"=""} ("错误输出")) -> ("Name"=w36:string)  [unwired: 2 out]
  n284 = String To Path(string=w31) -> (path=w28:path)
  n285 = Open VI Reference(type specifier VI Refnum (for type only)=refnum<vi> refnum, vi path=w36, options=128 ("选项")) -> (vi reference=w38:refnum<vi>, error out=w40:errorcluster)  [unwired: 3 in]
  n286 = Build Path(base path=w28, name or relative path=w34) -> (appended path=w4:path)
  n287 = call-by-ref "?"(reference=w38, error in=w40) -> (reference out=w42:refnum<vi>, error out=w41:errorcluster)  [unwired: 12 in]
  n288 = global read "多参数全局变量.vi" "TCP Connection Count"() -> (w5:u32)
  n289 = Close Reference(reference=w42, error in (no error)=w41) -> ()  [unwired: 1 out]
  n290 = case shown="1, 默认" w5 {
    tunnel: w4 -> [w425 w428]
    tunnel: [w425 w427] -> w2
    tunnel: [_ w426] -> w3
    frame 0 {
    }
    frame 1, Default {
      n291 = call <vilib>:"Check if File or Folder Exists.vi"("path"=w428) -> ("file or folder exists?"=w426:bool, "dup path"=w427:path)  [unwired: 8 in, 1 out]
    }
  }
  n292 = case shown="假" w3 {
    tunnel: w2 -> [_ w432]
    tunnel: [w430 w432] -> w7
    tunnel: w34 -> [w429 _]
    frame False {
      # "本地文件地址"
      n293 = call <vilib>:"Application Directory.vi"() -> ("Application Directory"=w431:path)
      n294 = Build Path(base path=w431, name or relative path=w429) -> (appended path=w430:path)
    }
    frame True {
      # "网络共享地址"
    }
  }
  n295 = global write "多参数全局变量.vi" "配置文件 path"(w7) -> ()
  n296 = Equal?(x="编号", y="") -> (x = y?=w17:bool)
  n297 = call <vilib>:"Open Config Data.vi"("configuration file path"=w7) -> ("error out"=w47:errorcluster, "refnum"=w48:T19)  [unwired: 8 in, 1 out]
  n298 = Select(t="1", s=w17, f="编号") -> (s? t:f=w15:string)
  n299 = global write "多参数全局变量.vi" "多参数编号"(w15) -> ()
  n300 = while {
    stop <- FALSE stop-if-true
    n301 = Wait (ms)(milliseconds to wait=u32 1000 ("等待时间（毫秒）")) -> ()  [unwired: 1 out]
    n302 = global read "系统设置全局变量.vi" "三级权限"() -> (w436:bool)
    n303 = Select(t=T12."Enabled" ("禁用"), s=w436, f=T12."Disabled and Grayed Out" ("禁用")) -> (s? t:f=w433:T12)
    n304 = property on="设置" class="Bool"("DisabledEnum"=w433) -> ()  [unwired: 2 in, 2 out]
  }
  n305 = vi-ref "断电保存变量.vi"() -> (w44:refnum<vi>)
  n306 = case shown="\"假\", 默认" w15 {
    tunnel: [TRUE ("可见") FALSE ("可见")] -> w27
    frame "假", Default {
    }
    frame "001" {
    }
  }
  n307 = Concatenate Strings("MPresource" ("名称（未命名）"), w15) -> (w55:string)
  n308 = call <userlib>:"Read Panel from INI__ogtk.vi"("error in (no error)"=w47, "VI ref"=w44, "refnum"=w48) -> ("error out"=w45:errorcluster, "refnum out"=w46:T19)  [unwired: 7 in]
  n309 = Concatenate Strings("MPP" ("名称（未命名）"), w15) -> (w56:string)
  n310 = call <vilib>:"Close Config Data.vi"("error in (no error)"=w45, "refnum"=w46) -> ("error out"=w8:errorcluster)  [unwired: 8 in, 1 out]
  n311 = Obtain Queue(name (unnamed)=w55, element data type="" ("名称（未命名）")) -> (queue out=w51:refnum<queue>)  [unwired: 3 in, 2 out]
  n312 = property on="窗格" class="Pane"("Origin"=T3 {"Horizontal"=0, "Vertical"=0} ("原点")) -> (error out=w63:errorcluster)  [unwired: 2 in, 1 out]
  n313 = Read from Text File(file (use dialog)=w7, error in=w8) -> (error out=w6:errorcluster)  [unwired: 2 in, 3 out]
  n314 = Obtain Notifier(name (unnamed)=w56, notification data type=FALSE) -> (notifier out=w59:refnum<notifier>)  [unwired: 2 in, 2 out]
  n315 = Enqueue Element(queue=w51, element="open" ("元素")) -> (queue out=w50:refnum<queue>)  [unwired: 2 in, 2 out]
  n316 = while {
    tunnel: w50 -> [w442]
    tunnel: w6 -> [_]
    stop <- FALSE stop-if-true
    n317 = Dequeue Element(queue=w442) -> (element=w441:string)  [unwired: 2 in, 3 out]
    n318 = case shown="\"open\"" w441 {
      tunnel: [_ w453 w463] -> _
      tunnel: [_ w444 _] -> _
      frame "假", Default {
      }
      frame "open" {
        n319 = global read "多参数全局变量.vi" "MB session in 电导率"() -> (w448:refnum<class "MB_Master.lvclass">)
        n320 = global read "断电保存变量.vi" "电导率串口"() -> (w446:refnum<visa-resource-name>)
        n321 = global read "断电保存变量.vi" "连接方式"() -> (w450:u16)
        n322 = call "close MB.vi"("MB session in"=w448) -> ("error out"=w445:errorcluster)  [unwired: 10 in]
        n323 = global read "多参数全局变量.vi" "MB session in"() -> (w458:refnum<class "MB_Master.lvclass">)
        n324 = global read "断电保存变量.vi" "Port"() -> (w452:u16)
        n325 = global read "断电保存变量.vi" "IP"() -> (w451:string)
        n326 = call "open MB.vi"("Port (502)"=w452, "IP Address"=w451, "MODE"=w450, "error in (no error)"=w445, "Serial Config"=T20 {"baud rate (bps)"=9600, "stop bits"=10, "parity"=0, "flow control"=0, "timeout"=1000, "retries"=1}, "VISA资源名称"=w446) -> ("error out"=w444:errorcluster, "MB session out"=w449:refnum<class "MB_Master.lvclass">)  [unwired: 4 in]
        n327 = global read "断电保存变量.vi" "VISA资源名称"() -> (w460:refnum<visa-resource-name>)
        n328 = global write "多参数全局变量.vi" "MB session in 电导率"(w449) -> ()
        n329 = global read "断电保存变量.vi" "连接方式"() -> (w456:u16)
        n330 = call "close MB.vi"("MB session in"=w458) -> ("error out"=w461:errorcluster)  [unwired: 10 in]
        n331 = global read "断电保存变量.vi" "Port"() -> (w454:u16)
        n332 = global read "断电保存变量.vi" "IP"() -> (w455:string)
        n333 = call "open MB.vi"("Port (502)"=w454, "IP Address"=w455, "MODE"=w456, "error in (no error)"=w461, "Serial Config"=T20 {"baud rate (bps)"=9600, "stop bits"=10, "parity"=0, "flow control"=0, "timeout"=1000, "retries"=1}, "VISA资源名称"=w460) -> ("error out"=w453:errorcluster, "MB session out"=w457:refnum<class "MB_Master.lvclass">)  [unwired: 4 in]
        n334 = global write "多参数全局变量.vi" "MB session in"(w457) -> ()
      }
      frame "close" {
        n335 = global read "多参数全局变量.vi" "MB session in"() -> (w462:refnum<class "MB_Master.lvclass">)
        n336 = call "close MB.vi"("MB session in"=w462) -> ("error out"=w463:errorcluster)  [unwired: 10 in]
      }
    }
  }
  n337 = while {
    tunnel: [w471] -> _
    shift-right: [w464] -> _
    shift-left: _ -> [w469]
    tunnel: w6 -> [w466]
    stop <- FALSE stop-if-true
    n338 = Wait (ms)(milliseconds to wait=u32 1000 ("等待时间（毫秒）")) -> ()  [unwired: 1 out]
    n339 = global read "多参数全局变量.vi" "配置文件 path"() -> (w465:path)
    n340 = File/Directory Info(path=w465, error in=w466) -> (last mod=w464:timestamp, error out=w467:errorcluster)  [unwired: 5 out]
    n341 = Not Equal?(x=w464, y=w469) -> (x != y?=w468:bool)
    n342 = case shown="真" w468 {
      tunnel: [w473 w481] -> w471
      tunnel: w467 -> [w473 w480]
      tunnel: w465 -> [_ w474]
      frame False {
      }
      frame True {
        # "文件发生改变进行更新"
        n343 = call <vilib>:"Open Config Data.vi"("error in (no error)"=w480, "configuration file path"=w474) -> ("error out"=w479:errorcluster, "refnum"=w478:T19)  [unwired: 7 in, 1 out]
        n344 = vi-ref "断电保存变量.vi"() -> (w475:refnum<vi>)
        n345 = call <userlib>:"Read Panel from INI__ogtk.vi"("error in (no error)"=w479, "VI ref"=w475, "refnum"=w478) -> ("error out"=w477:errorcluster, "refnum out"=w476:T19)  [unwired: 7 in]
        n346 = call <vilib>:"Close Config Data.vi"("error in (no error)"=w477, "refnum"=w476) -> ("error out"=w481:errorcluster)  [unwired: 8 in, 1 out]
      }
    }
  }
  n347 = while {
    tunnel: w50 -> [w483]
    stop <- FALSE stop-if-true
    # "断线重连"
    n348 = global read "断电保存变量.vi" "连接方式"() -> (w484:u16)
    n349 = Wait (ms)(milliseconds to wait=u32 10000 ("等待时间（毫秒）")) -> ()  [unwired: 1 out]
    n350 = case shown="1" w484 {
      tunnel: w483 -> [_ w487]
      frame 0, Default {
      }
      frame 1 {
        n351 = case shown="真" "自动断线重连" {
          tunnel: w487 -> [_ w490]
          frame False {
          }
          frame True {
            n352 = global read "多参数全局变量.vi" "MB session in"() -> (w489:refnum<class "MB_Master.lvclass">)
            n353 = property class="MB_Master"(reference=w489) -> ("Properties:Session Valid"=w488:bool)  [unwired: 1 in, 2 out]
            n354 = case shown="假" w488 {
              tunnel: w490 -> [w491 _]
              frame False {
                n355 = Flush Queue(queue=w491) -> (queue out=w493:refnum<queue>)  [unwired: 1 in, 2 out]
                n356 = Enqueue Element(queue=w493, element="open" ("元素")) -> ()  [unwired: 2 in, 3 out]
              }
              frame True {
              }
            }
          }
        }
      }
    }
  }
  n357 = property on="编号" class="Str"("Visible"=w27) -> ()  [unwired: 2 in, 2 out]
  n358 = while {
    tunnel: w63 -> [_]
    tunnel: w59 -> [w495]
    tunnel: w50 -> [w494]
    stop <- FALSE stop-if-true
    n359 = event shown="[11] \"设置\": 值改变" {
      selector: _ -> [_ _ _ _ _ _ _ _ _ _ _ _ _ _ _ _ _ _ _ _ _ _ _ _]
      dyn-events: _ -> [_ _ _ _ _ _ _ _ _ _ _ _ _ _ _ _ _ _ _ _ _ _ _ _]
      timeout: _ -> [_ _ _ _ _ _ _ _ _ _ _ _ _ _ _ _ _ _ _ _ _ _ _ _]
      tunnel: w495 -> [_ _ _ _ _ _ _ _ _ _ w597 _ _ _ _ _ _ _ _ _ _ _ _ _]
      tunnel: w494 -> [_ _ _ _ _ _ _ _ _ _ _ _ _ _ w637 _ _ _ _ _ _ _ _ _]
      event Timeout {
        n360 = event-data() -> ()  [unwired: 1 in, 3 out]
      }
      event "水样稳定时间", "水样保存组数": Mouse Down {
        n361 = event-data() -> ("CtlRef"=w497:refnum<vi>)  [unwired: 1 in, 5 out]
        n362 = property class="DigNum (严格)"(reference=w497) -> (reference out=w500:refnum<vi>, "Value"=w499:dbl)  [unwired: 1 in, 1 out]
        n363 = call "数字键盘.vi"("OldNumber"=w499) -> ("NewNumber"=w498:dbl)  [unwired: 1 in]
        n364 = property class="DigNum (严格)"(reference=w500, "Val(Sgnl)"=w498) -> ()  [unwired: 1 in, 2 out]
      }
      event "pH探头选择", "DO探头选择", "电导率探头选择", "浊度探头选择", "叶绿素a探头选择", "藻密度探头选择", "ORP探头选择": Value Change {
        n365 = event-data() -> ("CtlRef"=w501:refnum<vi>, "NewVal"=w502:u16)  [unwired: 1 in, 4 out]
        n366 = Two Button Dialog(message="请再次确认修改的型号是否与实际匹配，否则将导致通讯异常，并且此操作将终止所有正在校准的参数！" ("消息")) -> (T button?=w503:bool)  [unwired: 2 in]
        n367 = case shown="真" w503 {
          tunnel: w502 -> [_ w506]
          tunnel: w501 -> [_ w505]
          frame False {
          }
          frame True {
            n368 = flat-sequence {
              tunnel: w506 -> [w507]
              tunnel: w505 -> [w511]
              frame #0 {
                n369 = property class="Ring (严格)"(reference=w511) -> ("Label.Text"=w510:string)  [unwired: 1 in, 2 out]
                n370 = global read "断电保存变量.vi" "探头选择"() -> (w509:T13)
                n371 = global read "多参数全局变量.vi" "校准VI引用句柄"() -> (w512:T21)
                n372 = case shown="\"ORP探头选择\"" w510 {
                  tunnel: w509 -> [w514 w517 w520 w523 w526 w529 w532 w535]
                  tunnel: [w514 w516 w519 w522 w525 w528 w531 w534] -> w508
                  tunnel: w507 -> [_ w515 w518 w521 w524 w527 w530 w533]
                  frame Default {
                  }
                  frame "pH探头选择" {
                    n373 = Bundle By Name(cluster=w517, "pH探头选择"=w515) -> (w516:T13)
                  }
                  frame "电导率探头选择" {
                    n374 = Bundle By Name(cluster=w520, "电导率探头选择"=w518) -> (w519:T13)
                  }
                  frame "DO探头选择" {
                    n375 = Bundle By Name(cluster=w523, "DO探头选择"=w521) -> (w522:T13)
                  }
                  frame "浊度探头选择" {
                    n376 = Bundle By Name(cluster=w526, "浊度探头选择"=w524) -> (w525:T13)
                  }
                  frame "叶绿素a探头选择" {
                    n377 = Bundle By Name(cluster=w529, "叶绿素a探头选择"=w527) -> (w528:T13)
                  }
                  frame "蓝绿藻探头选择" {
                    n378 = Bundle By Name(cluster=w532, "蓝绿藻探头选择"=w530) -> (w531:T13)
                  }
                  frame "ORP探头选择" {
                    n379 = Bundle By Name(cluster=w535, "蓝绿藻探头选择"=w533) -> (w534:T13)
                  }
                }
                n380 = Cluster To Array(cluster=w512) -> (array=w513:refnum<vi>[])
                n381 = for {
                  tunnel: w513 -> [w537] mode=indexing
                  tunnel: [w536] -> _ mode=indexing
                  n382 = invoke class="VI" method="Abort VI"(reference=w537) -> (error out=w536:errorcluster)  [unwired: 2 in, 2 out]
                }
                n383 = global write "断电保存变量.vi" "探头选择"(w508) -> ()
              }
              frame #1 {
                n384 = call "配置文件保存.vi"() -> ()  [unwired: 12 in]
              }
            }
          }
        }
      }
      event "VISA资源名称", "pH", "DO", "Turb", "Cond", "Temp", "叶绿素a启用", "打开modbus", "藻密度", "连接方式", "自动断线重连", "ORP启用": Mouse Down {
        n385 = event-data() -> ()  [unwired: 1 in, 6 out]
        n386 = local read "密码锁"() -> (w538:bool)
        n387 = case shown="假" w538 {
          frame False {
            n388 = One Button Dialog(message="当前操作权限不足,请提升权限!!!" ("消息")) -> ()  [unwired: 1 in, 1 out]
          }
          frame True {
          }
        }
      }
      event "IP": Mouse Down {
        n389 = event-data() -> ("CtlRef"=w541:refnum<vi>)  [unwired: 1 in, 7 out]
        n390 = property on="IP" class="Str"() -> ("DisabledEnum"=w540:T12)  [unwired: 2 in, 2 out]
        n391 = case shown="\"Disabled and Grayed Out\"" w540 {
          tunnel: w541 -> [w545 _ _]
          frame "Enabled" {
            n392 = property class="Str"(reference=w545) -> (reference out=w544:refnum<vi>, "Value"=w543:string)  [unwired: 1 in, 1 out]
            n393 = call "字符键盘.vi"("Old String"=w543) -> ("String"=w542:string)  [unwired: 10 in]
            n394 = property class="Str"(reference=w544, "Val(Sgnl)"=w542) -> ()  [unwired: 1 in, 2 out]
          }
          frame "Disabled and Grayed Out" {
            n395 = One Button Dialog(message="关闭连接后才可设置!" ("消息")) -> ()  [unwired: 1 in, 1 out]
          }
          frame "Disabled", Default {
            n396 = One Button Dialog(message="当前操作权限不足,请提升权限!!!" ("消息")) -> ()  [unwired: 1 in, 1 out]
          }
        }
      }
      event "Port": Mouse Down {
        n397 = event-data() -> ("CtlRef"=w549:refnum<vi>)  [unwired: 1 in, 7 out]
        n398 = property on="Port" class="DigNum (严格)"() -> ("DisabledEnum"=w548:T12)  [unwired: 2 in, 2 out]
        n399 = case shown="\"Enabled\"" w548 {
          tunnel: w549 -> [w553 _ _]
          frame "Enabled" {
            n400 = property class="DigNum (严格)"(reference=w553) -> (reference out=w552:refnum<vi>, "Value"=w551:u16)  [unwired: 1 in, 1 out]
            n401 = call "数字键盘.vi"("OldNumber"=w551) -> ("NewNumber"=w550:dbl)  [unwired: 1 in]
            n402 = property class="DigNum (严格)"(reference=w552, "Val(Sgnl)"=w550) -> ()  [unwired: 1 in, 2 out]
          }
          frame "Disabled and Grayed Out" {
            n403 = One Button Dialog(message="关闭连接后才可设置!" ("消息")) -> ()  [unwired: 1 in, 1 out]
          }
          frame "Disabled", Default {
            n404 = One Button Dialog(message="当前操作权限不足,请提升权限!!!" ("消息")) -> ()  [unwired: 1 in, 1 out]
          }
        }
      }
      event "密码锁": Value Change {
        n405 = event-data() -> ("NewVal"=w556:bool)  [unwired: 1 in, 5 out]
        n406 = case shown="假" w556 {
          frame False {
            n407 = global write "多参数全局变量.vi" "权限"(enum16{"一级权限", "二级权限", "三级权限"}."一级权限" ("权限")) -> ()
          }
          frame True {
            n408 = call "数字键盘.vi"("显示样式"=u32 2) -> ("NewNumber"=w561:dbl)  [unwired: 1 in]
            n409 = case shown="23506" w561 {
              tunnel: ["密码错误,即将切换为一级权限!" ("Infoin") "密码正确,即将切换为二级权限!" ("Infoin") "密码正确,即将切换为三级权限!" ("Infoin")] -> w560
              tunnel: [u32 16711680 ("颜色盒") _ _] -> w559
              tunnel: [enum16{"一级权限", "二级权限", "三级权限"}."一级权限" ("权限") enum16{"一级权限", "二级权限", "三级权限"}."二级权限" ("权限") enum16{"一级权限", "二级权限", "三级权限"}."三级权限" ("权限")] -> w558
              frame 0, Default {
              }
              frame 666 {
              }
              frame 23506 {
              }
            }
            n410 = global write "多参数全局变量.vi" "权限"(w558) -> ()
            n411 = call "TimeLmtDialog.vi"("颜色盒"=w559, "Infoin"=w560) -> ()  [unwired: 10 in]
          }
        }
      }
      event "周期设置": Mouse Down {
        n412 = event-data() -> ()  [unwired: 1 in, 6 out]
        n413 = flat-sequence {
          frame #0 {
            n414 = global read "断电保存变量.vi" "定时控制输入"() -> (w571:T15)
            n415 = call "周期设置.vi"("定时控制输入"=w571) -> ("定时控制输出"=w570:T15)  [unwired: 10 in]
            n416 = global write "断电保存变量.vi" "定时控制输入"(w570) -> ()
          }
          frame #1 {
            n417 = call "配置文件保存.vi"() -> ()  [unwired: 12 in]
          }
        }
      }
      event "水样测试": Value Change {
        n418 = event-data() -> ()  [unwired: 1 in, 6 out]
        n419 = vi-ref "水样测试.vi"() -> (w574:refnum<vi>)
        n420 = property class="VI"(reference=w574) -> ("Name"=w578:string, "Exec.State"=w576:T16)  [unwired: 1 in, 2 out]
        n421 = Open VI Reference(type specifier VI Refnum (for type only)=refnum<vi> refnum, vi path=w578, options=128 ("选项")) -> (vi reference=w579:refnum<vi>)  [unwired: 3 in, 1 out]
        n422 = case shown="\"Idle\"" w576 {
          tunnel: [w580 w583] -> w575
          tunnel: w579 -> [w580 w582]
          tunnel: "hd" ("数据标记表") -> [_ w581]
          frame "Bad", Default {
          }
          frame "Idle" {
            n423 = call-by-ref "开始异步调用"(reference=w582, "数据标记表"=w581) -> (reference out=w583:refnum<vi>)  [unwired: 12 in, 1 out]
          }
        }
        n424 = Close Reference(reference=w575) -> ()  [unwired: 1 in, 1 out]
      }
      event "标样核查": Value Change {
        n425 = event-data() -> ()  [unwired: 1 in, 6 out]
        n426 = call "标样核查配置.vi"() -> ("确认输出"=w584:bool)  [unwired: 11 in]
        n427 = case shown="真" w584 {
          frame False {
          }
          frame True {
            n428 = vi-ref "标样核查.vi"() -> (w586:refnum<vi>)
            n429 = property class="VI"(reference=w586) -> ("Name"=w590:string, "Exec.State"=w588:T16)  [unwired: 1 in, 2 out]
            n430 = Open VI Reference(type specifier VI Refnum (for type only)=refnum<vi> refnum, vi path=w590, options=128 ("选项")) -> (vi reference=w591:refnum<vi>)  [unwired: 3 in, 1 out]
            n431 = case shown="\"Idle\"" w588 {
              tunnel: [w592 w594] -> w587
              tunnel: w591 -> [w592 w593]
              frame "Bad", Default {
              }
              frame "Idle" {
                n432 = call-by-ref "开始异步调用"(reference=w593) -> (reference out=w594:refnum<vi>)  [unwired: 13 in, 1 out]
              }
            }
            n433 = Close Reference(reference=w587) -> ()  [unwired: 1 in, 1 out]
          }
        }
      }
      event "停止": Value Change {
        w595 = u16 3 items=["空闲", "水样测试", "标样核查", "停止"] ("主副屏同步启动")
        n434 = event-data() -> ()  [unwired: 1 in, 6 out]
        n435 = Send Notification(notification=TRUE ("通知"), notifier=w597) -> ()  [unwired: 1 in, 2 out]
        n436 = global write "多参数全局变量.vi" "主副屏同步启动"(w595) -> ()
      }
      event "设置": Value Change {
        n437 = event-data() -> ()  [unwired: 1 in, 6 out]
        n438 = property on="窗格" class="Pane"("Origin"=T3 {"Horizontal"=0, "Vertical"=628} ("原点")) -> ()  [unwired: 2 in, 2 out]
      }
      event "仪器参数": Value Change {
        n439 = event-data() -> ()  [unwired: 1 in, 6 out]
        n440 = global read "断电保存变量.vi" "叶绿素参数"() -> (w599:T10)
        n441 = global read "断电保存变量.vi" "藻密度参数"() -> (w600:T10)
        n442 = global read "断电保存变量.vi" "电导率参数"() -> (w607:T10)
        n443 = global read "断电保存变量.vi" "溶解氧参数"() -> (w605:T10)
        n444 = global read "断电保存变量.vi" "ORP参数"() -> (w601:T10)
        n445 = global read "断电保存变量.vi" "水温参数"() -> (w608:T10)
        n446 = global read "断电保存变量.vi" "浊度参数"() -> (w606:T10)
        n447 = global read "断电保存变量.vi" "PH参数"() -> (w609:T10)
        n448 = Build Array(w609, w608, w607, w605, w606, w599, w600, w601) -> (w604:T22)
        n449 = call "仪器参数设置.vi"("仪器参数设置输入"=w604) -> ("确定"=w603:bool, "仪器参数设置输出"=w602:T22)  [unwired: 9 in]
        n450 = case shown="真" w603 {
          tunnel: w602 -> [_ w610]
          frame False {
          }
          frame True {
            n451 = flat-sequence {
              tunnel: w610 -> [w619]
              frame #0 {
                n452 = Index Array(array=w619) -> (element #1=w617:T10, element #2=w616:T10, element #3=w614:T10, element #4=w615:T10, element #5=w618:T10, element #6=w613:T10, element #7=w611:T10, element #8=w612:T10)  [unwired: 8 in]
                n453 = global write "断电保存变量.vi" "叶绿素参数"(w613) -> ()
                n454 = global write "断电保存变量.vi" "藻密度参数"(w611) -> ()
                n455 = global write "断电保存变量.vi" "PH参数"(w617) -> ()
                n456 = global write "断电保存变量.vi" "水温参数"(w616) -> ()
                n457 = global write "断电保存变量.vi" "电导率参数"(w614) -> ()
                n458 = global write "断电保存变量.vi" "溶解氧参数"(w615) -> ()
                n459 = global write "断电保存变量.vi" "浊度参数"(w618) -> ()
                n460 = global write "断电保存变量.vi" "ORP参数"(w612) -> ()
              }
              frame #1 {
                n461 = call "配置文件保存.vi"() -> ()  [unwired: 12 in]
              }
            }
          }
        }
      }
      event "pH", "DO", "Turb", "Cond", "Temp", "叶绿素a启用", "藻密度", "VISA资源名称", "连接方式", "IP", "Port", "自动断线重连", "水样稳定时间", "ORP启用", "电导率串口", "水样保存组数": Value Change {
        n462 = event-data() -> ()  [unwired: 1 in, 6 out]
        n463 = flat-sequence {
          frame #0 {
            n464 = global write "断电保存变量.vi" "IP"("IP") -> ()
            n465 = global write "断电保存变量.vi" "藻密度"("藻密度") -> ()
            n466 = global write "断电保存变量.vi" "连接方式"("连接方式") -> ()
            n467 = global write "断电保存变量.vi" "Temp"("Temp") -> ()
            n468 = global write "断电保存变量.vi" "DO"("DO") -> ()
            n469 = global write "断电保存变量.vi" "Turb"("Turb") -> ()
            n470 = global write "断电保存变量.vi" "Port"("Port") -> ()
            n471 = global write "断电保存变量.vi" "pH"("pH") -> ()
            n472 = global write "断电保存变量.vi" "orp"("ORP启用") -> ()
            n473 = global write "断电保存变量.vi" "Cond"("Cond") -> ()
            n474 = global write "断电保存变量.vi" "叶绿素a启用"("叶绿素a启用") -> ()
            n475 = global write "断电保存变量.vi" "VISA资源名称"("VISA资源名称") -> ()
            n476 = global write "断电保存变量.vi" "水样稳定时间"("水样稳定时间") -> ()
            n477 = global write "断电保存变量.vi" "电导率串口"("电导率串口") -> ()
            n478 = local read "自动断线重连"() -> (w624:bool)
            n479 = global write "断电保存变量.vi" "水样测试组数"("水样保存组数") -> ()
            n480 = global write "断电保存变量.vi" "自动断线重连"(w624) -> ()
          }
          frame #1 {
            n481 = call "配置文件保存.vi"() -> ()  [unwired: 12 in]
          }
          frame #2 {
          }
        }
      }
      event "打开modbus": Value Change {
        n482 = event-data() -> ()  [unwired: 1 in, 6 out]
        n483 = global read "多参数全局变量.vi" "MB session in"() -> (w642:refnum<class "MB_Master.lvclass">)
        n484 = Flush Queue(queue=w637) -> (queue out=w636:refnum<queue>)  [unwired: 1 in, 2 out]
        n485 = property class="MB_Master"(reference=w642) -> ("Properties:Session Valid"=w641:bool)  [unwired: 1 in, 2 out]
        n486 = Select(t="close" ("元素"), s=w641, f="open" ("元素")) -> (s? t:f=w638:string)
        n487 = Enqueue Element(queue=w636, element=w638) -> ()  [unwired: 2 in, 3 out]
      }
      event "探头校正返回", "设置页返回": Value Change {
        n488 = event-data() -> ()  [unwired: 1 in, 6 out]
        n489 = property on="窗格" class="Pane"("Origin"=T3 {"Horizontal"=0, "Vertical"=0} ("原点")) -> ()  [unwired: 2 in, 2 out]
      }
      event "探头校正", "校准选择.水温校准": Value Change {
        n490 = event-data() -> ()  [unwired: 1 in, 6 out]
        n491 = property on="窗格" class="Pane"("Origin"=T3 {"Horizontal"=1656, "Vertical"=0} ("原点")) -> ()  [unwired: 2 in, 2 out]
        n492 = vi-ref "水温校准.vi"() -> (w644:refnum<vi>)
        n493 = property class="VI"(reference=w644) -> (reference out=w646:refnum<vi>, "Exec.State"=w645:T16)  [unwired: 1 in, 1 out]
        n494 = case shown="\"Bad\", 默认" w645 {
          tunnel: [w650 w652] -> w648
          tunnel: w646 -> [w650 w651]
          frame "Bad", Default {
          }
          frame "Idle" {
            n495 = invoke class="VI" method="Run VI"(reference=w651, "Wait until done"=FALSE ("结束前等待"), "Auto Dispose Ref"=FALSE ("自动销毁引用")) -> (reference out=w652:refnum<vi>)  [unwired: 2 in, 4 out]
          }
        }
        n496 = invoke on="探头校准子面板" class="SubPnl" method="Remove VI"() -> (error out=w647:errorcluster)  [unwired: 3 in, 2 out]
        n497 = invoke on="探头校准子面板" class="SubPnl" method="Insert VI"(error in=w647, "VI Ref"=w648) -> ()  [unwired: 2 in, 4 out]
      }
      event "校准选择.pH校准": Value Change {
        n498 = event-data() -> ()  [unwired: 1 in, 6 out]
        n499 = global read "断电保存变量.vi" "探头选择"() -> (w660:T13)
        n500 = Unbundle By Name(w660) -> ("pH探头选择"=w659:u16)
        n501 = case shown="2" w659 {
          tunnel: [w664 w665 w666] -> w658
          frame 0, Default {
            n502 = vi-ref "斯坦道多参数.lvlib:禹山pH校准.vi"() -> (w664:refnum<vi>)
          }
          frame 1 {
            n503 = vi-ref "斯坦道多参数.lvlib:pH电极校准.vi"() -> (w665:refnum<vi>)
          }
          frame 2 {
            n504 = vi-ref "斯坦道多参数.lvlib:纳清pH电极校准.vi"() -> (w666:refnum<vi>)
          }
        }
        n505 = property class="VI"(reference=w658) -> (reference out=w662:refnum<vi>, "Exec.State"=w661:T16)  [unwired: 1 in, 1 out]
        n506 = case shown="\"Bad\", 默认" w661 {
          tunnel: w662 -> [w667 w671]
          tunnel: [w667 w668] -> w656
          frame "Bad", Default {
          }
          frame "Idle" {
            n507 = invoke class="VI" method="Run VI"(reference=w671, "Wait until done"=FALSE ("结束前等待"), "Auto Dispose Ref"=FALSE ("自动销毁引用")) -> (reference out=w668:refnum<vi>)  [unwired: 2 in, 4 out]
          }
        }
        n508 = global read "多参数全局变量.vi" "校准VI引用句柄"() -> (w657:T21)
        n509 = invoke on="探头校准子面板" class="SubPnl" method="Remove VI"() -> (error out=w663:errorcluster)  [unwired: 3 in, 2 out]
        n510 = invoke on="探头校准子面板" class="SubPnl" method="Insert VI"(error in=w663, "VI Ref"=w656) -> ()  [unwired: 2 in, 4 out]
        n511 = Bundle By Name(cluster=w657, "pH校准VI引用句柄"=w656) -> (w655:T21)
        n512 = global write "多参数全局变量.vi" "校准VI引用句柄"(w655) -> ()
      }
      event "校准选择.电导率校准": Value Change {
        n513 = event-data() -> ()  [unwired: 1 in, 6 out]
        n514 = global read "断电保存变量.vi" "探头选择"() -> (w677:T13)
        n515 = Unbundle By Name(w677) -> ("电导率探头选择"=w676:u16)
        n516 = case shown="2" w676 {
          tunnel: [w681 w682 w683] -> w675
          frame 0, Default {
            n517 = vi-ref "斯坦道多参数.lvlib:禹山电导率校准.vi"() -> (w681:refnum<vi>)
          }
          frame 1 {
            n518 = vi-ref "斯坦道多参数.lvlib:电导率电极校准.vi"() -> (w682:refnum<vi>)
          }
          frame 2 {
            n519 = vi-ref "斯坦道多参数.lvlib:纳清电导率电极校准.vi"() -> (w683:refnum<vi>)
          }
        }
        n520 = property class="VI"(reference=w675) -> (reference out=w679:refnum<vi>, "Exec.State"=w678:T16)  [unwired: 1 in, 1 out]
        n521 = case shown="\"Bad\", 默认" w678 {
          tunnel: [w684 w686] -> w672
          tunnel: w679 -> [w684 w685]
          frame "Bad", Default {
          }
          frame "Idle" {
            n522 = invoke class="VI" method="Run VI"(reference=w685, "Wait until done"=FALSE ("结束前等待"), "Auto Dispose Ref"=FALSE ("自动销毁引用")) -> (reference out=w686:refnum<vi>)  [unwired: 2 in, 4 out]
          }
        }
        n523 = global read "多参数全局变量.vi" "校准VI引用句柄"() -> (w674:T21)
        n524 = invoke on="探头校准子面板" class="SubPnl" method="Remove VI"() -> (error out=w680:errorcluster)  [unwired: 3 in, 2 out]
        n525 = Bundle By Name(cluster=w674, "COND校准VI引用句柄"=w672) -> (w673:T21)
        n526 = invoke on="探头校准子面板" class="SubPnl" method="Insert VI"(error in=w680, "VI Ref"=w672) -> ()  [unwired: 2 in, 4 out]
        n527 = global write "多参数全局变量.vi" "校准VI引用句柄"(w673) -> ()
      }
      event "校准选择.溶解氧校准": Value Change {
        n528 = event-data() -> ()  [unwired: 1 in, 6 out]
        n529 = global read "断电保存变量.vi" "探头选择"() -> (w694:T13)
        n530 = Unbundle By Name(w694) -> ("DO探头选择"=w693:u16)
        n531 = case shown="2" w693 {
          tunnel: [w698 w699 w700] -> w692
          frame 0, Default {
            n532 = vi-ref "斯坦道多参数.lvlib:禹山溶解氧校准.vi"() -> (w698:refnum<vi>)
          }
          frame 1 {
            n533 = vi-ref "斯坦道多参数.lvlib:溶解氧电极校准.vi"() -> (w699:refnum<vi>)
          }
          frame 2 {
            n534 = vi-ref "斯坦道多参数.lvlib:纳清DO电极校准.vi"() -> (w700:refnum<vi>)
          }
        }
        n535 = property class="VI"(reference=w692) -> (reference out=w696:refnum<vi>, "Exec.State"=w695:T16)  [unwired: 1 in, 1 out]
        n536 = case shown="\"Bad\", 默认" w695 {
          tunnel: [w701 w703] -> w689
          tunnel: w696 -> [w701 w702]
          frame "Bad", Default {
          }
          frame "Idle" {
            n537 = invoke class="VI" method="Run VI"(reference=w702, "Wait until done"=FALSE ("结束前等待"), "Auto Dispose Ref"=FALSE ("自动销毁引用")) -> (reference out=w703:refnum<vi>)  [unwired: 2 in, 4 out]
          }
        }
        n538 = global read "多参数全局变量.vi" "校准VI引用句柄"() -> (w691:T21)
        n539 = invoke on="探头校准子面板" class="SubPnl" method="Remove VI"() -> (error out=w697:errorcluster)  [unwired: 3 in, 2 out]
        n540 = invoke on="探头校准子面板" class="SubPnl" method="Insert VI"(error in=w697, "VI Ref"=w689) -> ()  [unwired: 2 in, 4 out]
        n541 = Bundle By Name(cluster=w691, "DO校准VI引用句柄"=w689) -> (w690:T21)
        n542 = global write "多参数全局变量.vi" "校准VI引用句柄"(w690) -> ()
      }
      event "校准选择.浊度校准": Value Change {
        n543 = event-data() -> ()  [unwired: 1 in, 6 out]
        n544 = global read "断电保存变量.vi" "探头选择"() -> (w711:T13)
        n545 = Unbundle By Name(w711) -> ("浊度探头选择"=w710:u16)
        n546 = case shown="2" w710 {
          tunnel: [w715 w716 w717] -> w709
          frame 0, Default {
            n547 = vi-ref "斯坦道多参数.lvlib:禹山浊度校准.vi"() -> (w715:refnum<vi>)
          }
          frame 1 {
            n548 = vi-ref "斯坦道多参数.lvlib:浊度电极校准.vi"() -> (w716:refnum<vi>)
          }
          frame 2 {
            n549 = vi-ref "斯坦道多参数.lvlib:纳清浊度电极校准.vi"() -> (w717:refnum<vi>)
          }
        }
        n550 = property class="VI"(reference=w709) -> (reference out=w713:refnum<vi>, "Exec.State"=w712:T16)  [unwired: 1 in, 1 out]
        n551 = case shown="\"Bad\", 默认" w712 {
          tunnel: [w718 w720] -> w706
          tunnel: w713 -> [w718 w719]
          frame "Bad", Default {
          }
          frame "Idle" {
            n552 = invoke class="VI" method="Run VI"(reference=w719, "Wait until done"=FALSE ("结束前等待"), "Auto Dispose Ref"=FALSE ("自动销毁引用")) -> (reference out=w720:refnum<vi>)  [unwired: 2 in, 4 out]
          }
        }
        n553 = global read "多参数全局变量.vi" "校准VI引用句柄"() -> (w708:T21)
        n554 = invoke on="探头校准子面板" class="SubPnl" method="Remove VI"() -> (error out=w714:errorcluster)  [unwired: 3 in, 2 out]
        n555 = invoke on="探头校准子面板" class="SubPnl" method="Insert VI"(error in=w714, "VI Ref"=w706) -> ()  [unwired: 2 in, 4 out]
        n556 = Bundle By Name(cluster=w708, "TURB校准VI引用句柄"=w706) -> (w707:T21)
        n557 = global write "多参数全局变量.vi" "校准VI引用句柄"(w707) -> ()
      }
      event "校准选择.叶绿素a校准": Value Change {
        n558 = event-data() -> ()  [unwired: 1 in, 6 out]
        n559 = global read "断电保存变量.vi" "探头选择"() -> (w727:T13)
        n560 = Unbundle By Name(w727) -> ("叶绿素a探头选择"=w726:u16)
        n561 = case shown="2" w726 {
          tunnel: [w732 _ w733] -> w728
          frame 0, Default {
            n562 = vi-ref "禹山叶绿素a校准.vi"() -> (w732:refnum<vi>)
          }
          frame 1 {
          }
          frame 2 {
            n563 = vi-ref "斯坦道多参数.lvlib:纳清叶绿素a电极校准.vi"() -> (w733:refnum<vi>)
          }
        }
        n564 = property class="VI"(reference=w728) -> (reference out=w730:refnum<vi>, "Exec.State"=w729:T16)  [unwired: 1 in, 1 out]
        n565 = case shown="\"Bad\", 默认" w729 {
          tunnel: [w734 w736] -> w723
          tunnel: w730 -> [w734 w735]
          frame "Bad", Default {
          }
          frame "Idle" {
            n566 = invoke class="VI" method="Run VI"(reference=w735, "Wait until done"=FALSE ("结束前等待"), "Auto Dispose Ref"=FALSE ("自动销毁引用")) -> (reference out=w736:refnum<vi>)  [unwired: 2 in, 4 out]
          }
        }
        n567 = global read "多参数全局变量.vi" "校准VI引用句柄"() -> (w725:T21)
        n568 = invoke on="探头校准子面板" class="SubPnl" method="Remove VI"() -> (error out=w731:errorcluster)  [unwired: 3 in, 2 out]
        n569 = invoke on="探头校准子面板" class="SubPnl" method="Insert VI"(error in=w731, "VI Ref"=w723) -> ()  [unwired: 2 in, 4 out]
        n570 = Bundle By Name(cluster=w725, "CHLA校准VI引用句柄"=w723) -> (w724:T21)
        n571 = global write "多参数全局变量.vi" "校准VI引用句柄"(w724) -> ()
      }
      event "校准选择.藻密度校准": Value Change {
        n572 = event-data() -> ()  [unwired: 1 in, 6 out]
        n573 = global read "断电保存变量.vi" "探头选择"() -> (w743:T13)
        n574 = Unbundle By Name(w743) -> ("蓝绿藻探头选择"=w742:u16)
        n575 = case shown="2" w742 {
          tunnel: [_ w748] -> w744
          frame 0, Default {
          }
          frame 2 {
            n576 = vi-ref "斯坦道多参数.lvlib:纳清蓝绿藻电极校准.vi"() -> (w748:refnum<vi>)
          }
        }
        n577 = property class="VI"(reference=w744) -> (reference out=w746:refnum<vi>, "Exec.State"=w745:T16)  [unwired: 1 in, 1 out]
        n578 = case shown="\"Bad\", 默认" w745 {
          tunnel: [w749 w751] -> w739
          tunnel: w746 -> [w749 w750]
          frame "Bad", Default {
          }
          frame "Idle" {
            n579 = invoke class="VI" method="Run VI"(reference=w750, "Wait until done"=FALSE ("结束前等待"), "Auto Dispose Ref"=FALSE ("自动销毁引用")) -> (reference out=w751:refnum<vi>)  [unwired: 2 in, 4 out]
          }
        }
        n580 = global read "多参数全局变量.vi" "校准VI引用句柄"() -> (w741:T21)
        n581 = invoke on="探头校准子面板" class="SubPnl" method="Remove VI"() -> (error out=w747:errorcluster)  [unwired: 3 in, 2 out]
        n582 = invoke on="探头校准子面板" class="SubPnl" method="Insert VI"(error in=w747, "VI Ref"=w739) -> ()  [unwired: 2 in, 4 out]
        n583 = Bundle By Name(cluster=w741, "BGA校准VI引用句柄"=w739) -> (w740:T21)
        n584 = global write "多参数全局变量.vi" "校准VI引用句柄"(w740) -> ()
      }
      event "校准选择.ORP校准": Value Change {
        n585 = event-data() -> ()  [unwired: 1 in, 6 out]
        n586 = global read "断电保存变量.vi" "探头选择"() -> (w758:T13)
        n587 = Unbundle By Name(w758) -> ("orp探头选择"=w757:u16)
        n588 = case shown="1" w757 {
          tunnel: [_ w763] -> w759
          frame 0, Default {
          }
          frame 1 {
            n589 = vi-ref "斯坦道多参数.lvlib:ORP电极校准.vi"() -> (w763:refnum<vi>)
          }
        }
        n590 = property class="VI"(reference=w759) -> (reference out=w761:refnum<vi>, "Exec.State"=w760:T16)  [unwired: 1 in, 1 out]
        n591 = case shown="\"Bad\", 默认" w760 {
          tunnel: [w764 w766] -> w754
          tunnel: w761 -> [w764 w765]
          frame "Bad", Default {
          }
          frame "Idle" {
            n592 = invoke class="VI" method="Run VI"(reference=w765, "Wait until done"=FALSE ("结束前等待"), "Auto Dispose Ref"=FALSE ("自动销毁引用")) -> (reference out=w766:refnum<vi>)  [unwired: 2 in, 4 out]
          }
        }
        n593 = global read "多参数全局变量.vi" "校准VI引用句柄"() -> (w756:T21)
        n594 = invoke on="探头校准子面板" class="SubPnl" method="Remove VI"() -> (error out=w762:errorcluster)  [unwired: 3 in, 2 out]
        n595 = Bundle By Name(cluster=w756, "ORP校准VI引用句柄"=w754) -> (w755:T21)
        n596 = invoke on="探头校准子面板" class="SubPnl" method="Insert VI"(error in=w762, "VI Ref"=w754) -> ()  [unwired: 2 in, 4 out]
        n597 = global write "多参数全局变量.vi" "校准VI引用句柄"(w755) -> ()
      }
    }
  }
